vi "Sequence.vi"(8 "error in (no error)":errorcluster, 11 "Message Queues in":T65) -> (0 "error out":errorcluster)   [LabVIEW 2018, in "Sequencing Library.lvlib"]
uses:
  Sequencing Library.lvlib
  Main/Main Queue Cluster.ctl
  support/Message Queue/Message Cluster.ctl
  Drag and Drop/State Cluster.ctl
  Drag and Drop/Thumbnail Cluster.ctl
  Drag and Drop/Object Cluster.ctl
  <vilib>/Utility/miscctls.llb/LVRectTypeDef.ctl
  Drag and Drop/Object Type Enum.ctl
  <vilib>/Utility/miscctls.llb/LVPositionTypeDef.ctl
  Config Module/Controls/Main Config Cluster.ctl
  OPC/OPC Module Config.ctl
  Scale Module Folder/Measure Instrument/State Enum.ctl
  <vilib>/Utility/miscctls.llb/LVPoint32TypeDef.ctl
  OPC/OPC Settings.ctl
  OPC/Variable Data Cluster.ctl
  <vilib>/OPCUA/controls/NodeId.ctl
  <vilib>/OPCUA/controls/OPC UA StatusCode.ctl
  <vilib>/OPCUA/controls/Subscription ID.ctl
  <vilib>/OPCUA/controls/OPC UA Client Refnum.ctl
  <vilib>/OPCUA/controls/Subscription Data Change.ctl
  <vilib>/OPCUA/controls/Data Type.ctl
  Feed Module/Controls/Feed Module Config Cluster.ctl
  Feed Module/Controls/Feed Module Settings Cluster.ctl
  Ismatec ISM 831C/Controls/Ismatech Settings Cluster.ctl
  Masterflex 7550-30/Controls/Settings Cluster.ctl
  Mettler Toledo/Controls/Settings Cluster.ctl
  Bronkhorst M13 Flow Meter/Settings Cluster.ctl
  Measure Instrument/PID 2 Parameters Cluster.ctl
  Measure Instrument/PID Input Enum.ctl
  Measure Instrument/PID 2 Output Enum.ctl
  Tacmina QI/Tacmina QI DAQ Setting.ctl
  KNF Pump/Settings Cluster plus SIMDOS.ctl
  ASIA Pump/Pump Settings.ctl
  VICI M50 Party Mode/Settings Cluster.ctl
  FLOM Pump/Settings Cluster.ctl
  SSI PR Class/SSI PR or LD Settings Cluster.ctl
  Masterflex 75211/Masterflex 75211 DAQ Setting.ctl
  SSI PR Class/SSI P40 Settings Cluster.ctl
  TT Module/Controls/TT Module Config Cluster.ctl
  Tag VIs/Numeric Alarm Settings Cluster.ctl
  Acquisition/Hardware Configuration.ctl
  Acquisition/Task Cluster.ctl
  PT Module/Controls/PT Module Config Cluster.ctl
  Scale Module Folder/Feed Module/Controls/Scale Module Config Cluster.ctl
  Scale Module Folder/Feed Module/Controls/Scale Module Settings Cluster.ctl
  Pump Module Folder/Pump Module Config Cluster.ctl
  Pump Module Folder/Pump Module Settings Cluster.ctl
  LabJack Module/Controls/U3 Module Config Cluster.ctl
  Decoration Module/Decoration Module Config Cluster.ctl
  Flow Module Folder/Feed Module/Controls/Flow Module Config Cluster.ctl
  Flow Module Folder/Feed Module/Controls/Flow Module Settings Cluster.ctl
  TCU Module/TCU Module Folder/TCU Module Config Cluster.ctl
  TCU Module/TCU Module Folder/TCU Module Settings Cluster.ctl
  TCU Module/TCU Module Folder/Measure Instrument/Output Devices.ctl
  Huber TCU/Huber Settings.ctl
  Lauda Integral XT-150 TCU/Lauda Settings.ctl
  Julabo Type 1 TCU/Julabo Type 1 TCU Folder/Julabo FP-50 Settings.ctl
  Huber Unistat 410 TCU/Huber Unistat 410 RS485 Settings.ctl
  D-O Module Folder/Not Sure Where this is Used.ctl
  Squence Control.ctl
  D-O Module Folder/D-O Module Config Cluster.ctl
  D-O Module Folder/Valve Clusters.ctl
  D-O Module Folder/D-O Module Settings Cluster.ctl
  D-O Module Folder/D-O Device Settings Cluster.ctl
  VICI Electronic Actuator/VICI Electronic Actuator Settings.ctl
  Pressure Regulator Control Module/Pressure Regulator/Controls/4-20mA Module Config Cluster.ctl
  Pressure Regulator Control Module/Pressure Regulator/Controls/4-20mA Module Settings Cluster.ctl
  Pressure Transmitter/Pressure Transmitter Device Settings.ctl
  Pressure Reg Module/Pressure Regulator Device Settings.ctl
  Squence Update Cluster.ctl
  support/Message Queue/Enqueue Message (Single).vi
  support/Message Queue/Message Queue.lvlib
  support/Command Log VIs/Command Logging.lvlib
  Drag and Drop/Drag and Drop.lvlib
  Config Module/Config Module.lvlib
  TT Module/TT Module.lvlib
  Feed Module/Feed Module.lvlib
  Ismatec ISM 831C/Ismatec ISM 831C.lvlib
  Masterflex 7550-30/Masterflex 7550-30.lvlib
  Mettler Toledo/Mettler Toledo.lvlib
  Bronkhorst M13 Flow Meter/Bronkhorst M13 Flow Meter.lvlib
  Tacmina QI/Tacmina QI.lvlib
  KNF Pump/KNF SIMDOS.lvlib
  ASIA Pump.lvlib
  DAQ/DAQ.lvlib
  PT Module/PT Module.lvlib
  Scale Module Folder/Scale Module.lvlib
  Pump Module Folder/Pump Module.lvlib
  LabJack Module/U3 Module.lvlib
  Flow Module Folder/Flow Module.lvlib
  TCU Module/TCU Module Folder/TCU Module.lvlib
  Huber TCU/Huber Ministat 230 TCU.lvlib
  Lauda Integral XT-150 TCU/Lauda TCU.lvlib
  Julabo Type 1 TCU/Julabo Type 1 TCU Folder/Julabo Type FP-50 TCU.lvlib
  VICI M50 Party Mode/VICI M6 M50 Party Mode.lvlib
  D-O Module Folder/D-O Module.lvlib
  Pressure Transmitter/Pressure Transmitter Library.lvlib
  Pressure Regulator Control Module/Pressure Regulator/4-20mA Module.lvlib
  Pressure Reg Module/Pressure Regulator Library.lvlib
  FLOM Pump/FLOM Pump.lvlib
  SSI PR Class/SSI PR or LD Pump.lvlib
  OPC/OPC UA.lvlib
  Scale Module Folder/Measure Instrument/Scale Module Engine.lvlib
  D-O Module Folder/DIO Valve/VICI Electronic Actuator.lvlib
  Masterflex 75211/Masterflex 75211.lvlib
  SSI PR Class/SSI P40 Pump.lvlib
  Huber Unistat 410 TCU/Huber Unistat 410 TCU.lvlib
panel:
  out "Metrics:Code Size":u32
  out "Metrics:Total Data Size":u32
  out "Application:All VIs In Memory":string[](array[string])
  out "error out 2":errorcluster
  out "Process Name":string
  out "Queue Name":string
  out "Loop Variable":u32
  out "Step":i32
  out "Done":bool
  out "Output":T1 {"Main Config"."PR Module Configs"."Settings"."PID 2 Parameters"."output range"."output low" format="%.2f"; "Main Config"."PR Module Configs"."Settings"."PID 2 Parameters"."output range"."output high" min=0.0 max=100.0 format="%.2f"; "Main Config"."PR Module Configs"."Settings"."PID 2 Parameters"."PID gains"."derivative time (Td, min)" format="%.3f"; "Main Config"."PR Module Configs"."Settings"."PID 2 Parameters"."PID gains"."integral time (Ti, min)" format="%.3f"; "Main Config"."PR Module Configs"."Settings"."PID 2 Parameters"."PID gains"."proportional gain (Kc)" format="%.3f"; "Main Config"."Steps"."Control" items=["Pump %", "Setpoint"]; "Main Config"."TCU Module Configs"."Settings"."Huber Unistat 410 Settings"."Address" min=0 max=99 format="%02.0f"; "Main Config"."TCU Module Configs"."Settings"."Julabo FP-50 Settings"."Pump Power" min=0 max=8 step=1; "Main Config"."TCU Module Configs"."Settings"."Lauda Settings"."Pump Power" min=0 max=8 step=1; "Main Config"."Pump Module Configs"."Settings"."ASIA Pump C"."channel" min=0 max=1 step=1; "Main Config"."Pump Module Configs"."Settings"."Masterflex"."Pump Number" min=1.0 max=20.0 step=1.0; "Main Config"."Pump Module Configs"."Settings"."Ismatech"."Pump Number" min=1.0 max=20.0 step=1.0; "Main Config"."Feed Module Configs"."Settings"."output range"."output low" min=0.0 max=100.0 format="%.2f"; "Main Config"."Feed Module Configs"."Settings"."output range"."output high" format="%.2f"; "Main Config"."Feed Module Configs"."Settings"."PID 2 Parameters"."PID gains"."derivative time (Td, min)" format="%.3f"; "Main Config"."Feed Module Configs"."Settings"."PID 2 Parameters"."PID gains"."integral time (Ti, min)" format="%.3f"; "Main Config"."Feed Module Configs"."Settings"."PID 2 Parameters"."PID gains"."proportional gain (Kc)" format="%.3f"; "Main Config"."Feed Module Configs"."Settings"."ASIA Pump C"."channel" min=0 max=1 step=1; "Main Config"."Feed Module Configs"."Settings"."Ismatech"."Pump Number" min=1.0 max=20.0 step=1.0; "Main Config"."Feed Module Configs"."Settings"."Masterflex"."Pump Number" min=1.0 max=20.0 step=1.0}
  out "Intruction Cluster":T55 {"Control" items=["Setpoint", "Pump %"]}
  out "Paused":bool
  out "Stop":bool
  in  "Input":T1 {"Main Config"."PR Module Configs"."Settings"."PID 2 Parameters"."output range"."output low" format="%.2f"; "Main Config"."PR Module Configs"."Settings"."PID 2 Parameters"."output range"."output high" min=0.0 max=100.0 format="%.2f"; "Main Config"."PR Module Configs"."Settings"."PID 2 Parameters"."PID gains"."derivative time (Td, min)" format="%.3f"; "Main Config"."PR Module Configs"."Settings"."PID 2 Parameters"."PID gains"."integral time (Ti, min)" format="%.3f"; "Main Config"."PR Module Configs"."Settings"."PID 2 Parameters"."PID gains"."proportional gain (Kc)" format="%.3f"; "Main Config"."Steps"."Control" items=["Pump %", "Setpoint"]; "Main Config"."TCU Module Configs"."Settings"."Huber Unistat 410 Settings"."Address" min=0 max=99 format="%02.0f"; "Main Config"."TCU Module Configs"."Settings"."Julabo FP-50 Settings"."Pump Power" min=0 max=8 step=1; "Main Config"."TCU Module Configs"."Settings"."Lauda Settings"."Pump Power" min=0 max=8 step=1; "Main Config"."Pump Module Configs"."Settings"."ASIA Pump C"."channel" min=0 max=1 step=1; "Main Config"."Pump Module Configs"."Settings"."Masterflex"."Pump Number" min=1.0 max=20.0 step=1.0; "Main Config"."Pump Module Configs"."Settings"."Ismatech"."Pump Number" min=1.0 max=20.0 step=1.0; "Main Config"."Feed Module Configs"."Settings"."output range"."output low" min=0.0 max=100.0 format="%.2f"; "Main Config"."Feed Module Configs"."Settings"."output range"."output high" format="%.2f"; "Main Config"."Feed Module Configs"."Settings"."PID 2 Parameters"."PID gains"."derivative time (Td, min)" format="%.3f"; "Main Config"."Feed Module Configs"."Settings"."PID 2 Parameters"."PID gains"."integral time (Ti, min)" format="%.3f"; "Main Config"."Feed Module Configs"."Settings"."PID 2 Parameters"."PID gains"."proportional gain (Kc)" format="%.3f"; "Main Config"."Feed Module Configs"."Settings"."ASIA Pump C"."channel" min=0 max=1 step=1; "Main Config"."Feed Module Configs"."Settings"."Ismatech"."Pump Number" min=1.0 max=20.0 step=1.0; "Main Config"."Feed Module Configs"."Settings"."Masterflex"."Pump Number" min=1.0 max=20.0 step=1.0}
  # "Instrument Settings"
  # "Instrument Settings"
  # "Output Instruments"
  # "Flow Meter Settings"
  # "Output Instruments"
  # "Scale Settings"
  # "Output Instruments"
  # "Input Instruments"
  # "Instrument Settings"
  # "Instrument Settings"
  # "Output Instruments"
  # "Flow Meter Settings"
  # "Output Instruments"
  # "Scale Settings"
  # "Output Instruments"
  # "Input Instruments"
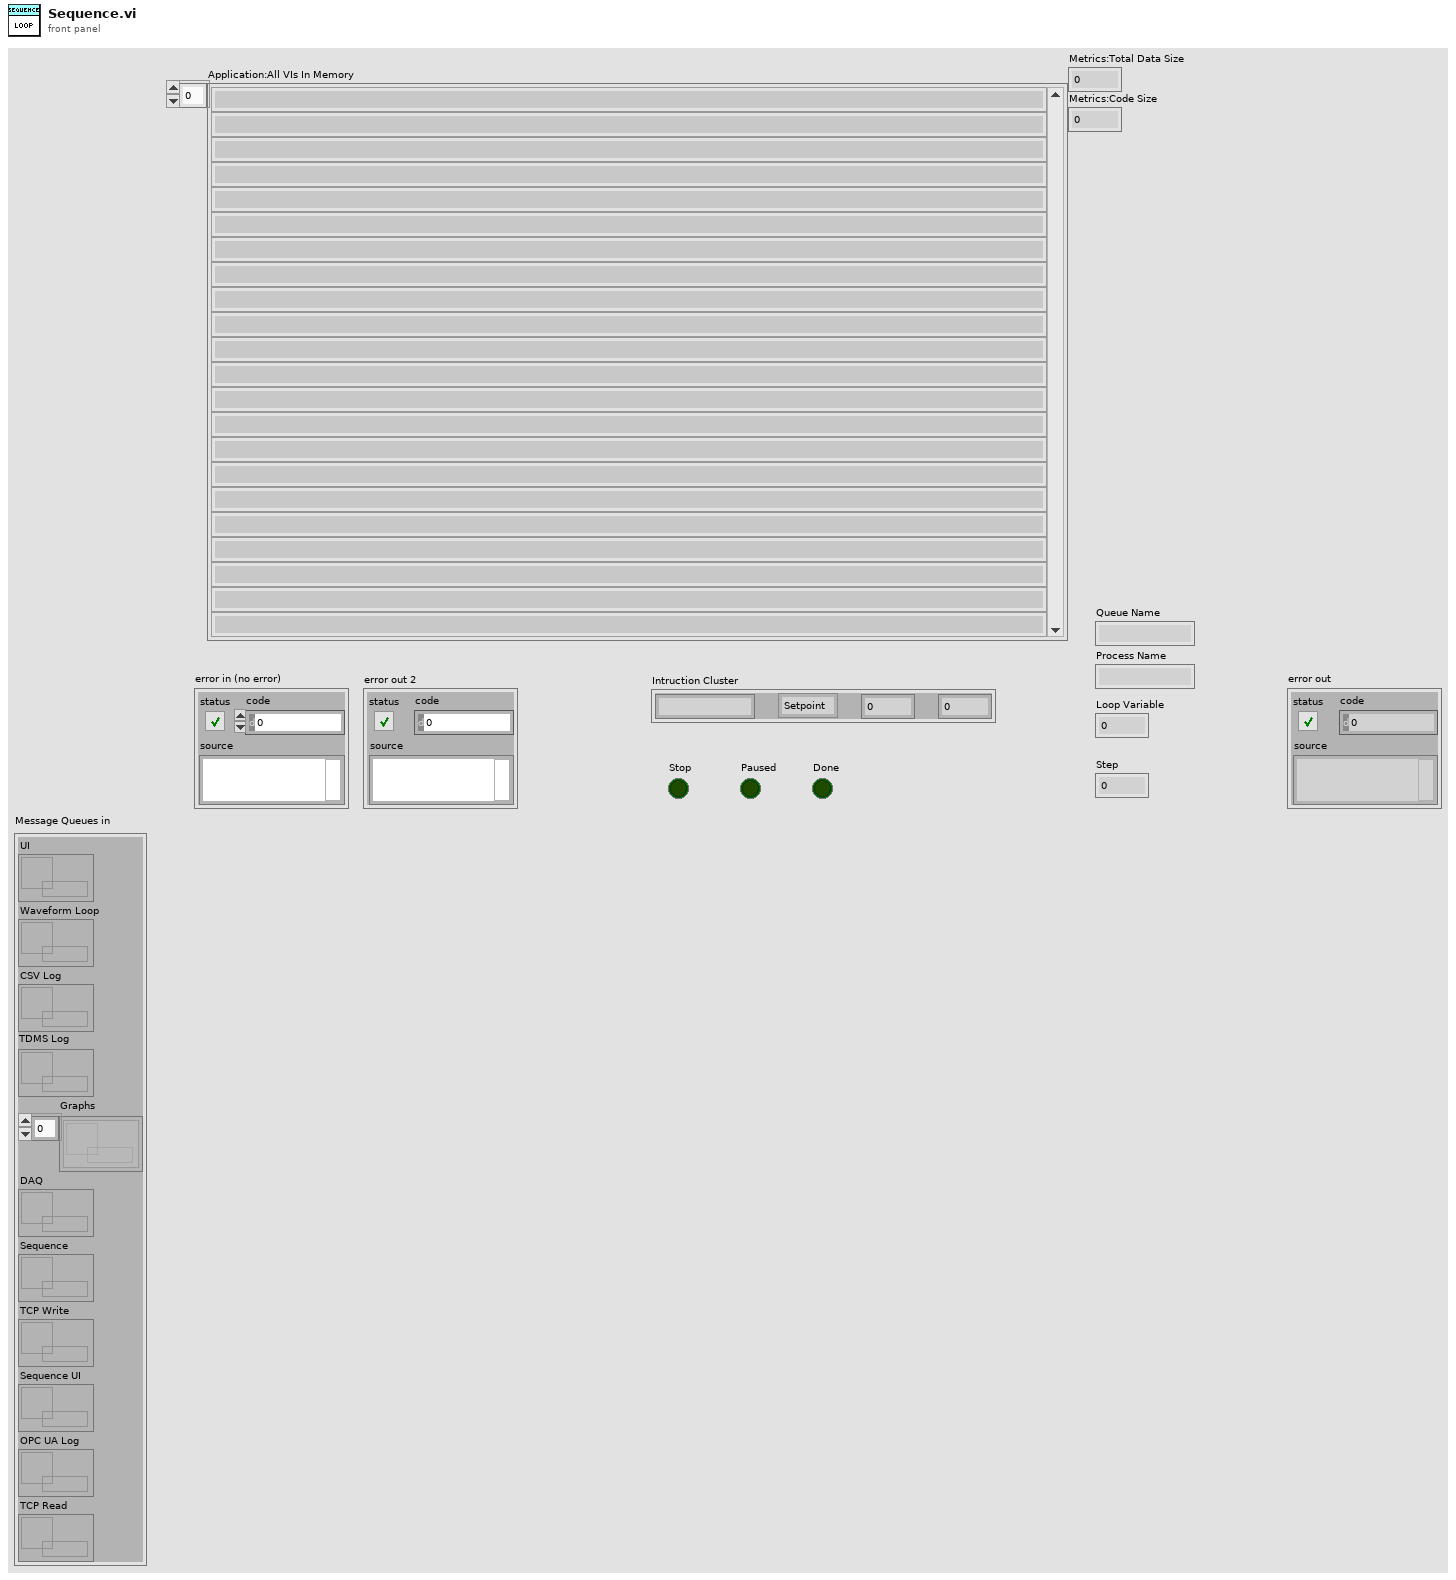
[diagram p1: front panel]
types:
  T1 = typedef "Drag and Drop.lvlib/State Cluster.ctl" = cluster{"VI refs":refnum<vi>[], "Queues":refnum<queue>[], "[Thumbnails]":T2[], "Drag Object Idx":i32, "[Objects]":T3[], "Active Object":i32, "Drop Offset":T6, "Process Name":string, "Main Config":T7, "Campaign Filepath":path, "Config Changed?":bool}
  T2 = typedef "Thumbnail Cluster.ctl" = cluster{"Path":path, "Rectangle":cluster{"left":i16, "top":i16, "right":i16, "bottom":i16}}
  T3 = typedef "Object Cluster.ctl" = cluster{"BMP Path":path, "Anchor Position":cluster{"X":i32, "Y":i32}, "Hot Spot":T4, "Type":T5, "Parameters":variant}
  T4 = typedef "LVRectTypeDef.ctl" = cluster{"Left":i16, "Top":i16, "Right":i16, "Bottom":i16}
  T5 = typedef "Object Type Enum.ctl" = enum16{"Icon", "Line", "Text", "Feed Module"}
  T6 = typedef "LVPositionTypeDef.ctl" = cluster{"Left":i32, "Top":i32}
  T7 = typedef "Config Module.lvlib/Main Config Cluster.ctl" = cluster{"Notebook":string, "Page":string, "OPC Module Configs":T8[], "Feed Module Configs":T17[], "Log File Path":path, "TT Module Configs":T34[], "DAQ Config":T36, "PT Module Configs":T38[], "Scale Module Configs":T39[], "Pump Module Configs":T41[], "U3 Module Configs":T43[], "Decoration Module Configs":T44[], "Flow Module Configs":T45[], "TCU Module Configs":T47[], "Steps":T54, "Abort":bool, "DO Module Configs":T56[], "PR Module Configs":T61[], "Cycle Period":dbl}
  T8 = typedef "OPC UA.lvlib/OPC Module Config.ctl" = cluster{"State":T9, "GUID":string, "Drop Coords":T10, "Configuration":T11, "First Iteration":bool, "Data":cluster{"Object Name":string, "Variable Array":T12[]}[], "Process Name":string, "Load Count":i32, "Log Started":bool, "subscription ID out":T15, "OPC UA client refnum out":T16, "Event Registration Refnum":refnum<event-registration>, "Start Time":timestamp, "Current Time":timestamp}
  T9 = typedef "Scale Module.lvlib/Scale Module Engine.lvlib/State Enum.ctl" = enum16{"Measuring", "Idle"}
  T10 = typedef "LVPoint32TypeDef.ctl" = cluster{"Horizontal":i32, "Vertical":i32}
  T11 = typedef "OPC UA.lvlib/OPC Settings.ctl" = cluster{"Cycle Period":dbl, "server endpoint URL":string, "security policy":cluster{"message mode":enum16{"None", "Sign", "Sign and Encrypt"}, "security":enum16{"Basic256", "Basic128Rsa15"}}, "Trust Any Server":bool}
  T12 = typedef "OPC UA.lvlib/Variable Data Cluster.ctl" = cluster{"node ID":T13, "browse name":string, "status":T14, "timestamp":timestamp, "value ":variant}
  T13 = typedef "NodeId.ctl" = string
  T14 = typedef "OPC UA StatusCode.ctl" = u32
  T15 = typedef "Subscription ID.ctl" = u32
  T16 = typedef "OPC UA Client Refnum.ctl" = refnum<k21>
  T17 = typedef "Feed Module.lvlib/Feed Module Config Cluster.ctl" = cluster{"GUID":string, "Drop Coords":T10, "Process Name":string, "Queue Name":string, "Settings":T18, "Settings Load Count":i32, "OP Load Count":i32}
  T18 = typedef "Feed Module.lvlib/Feed Module Settings Cluster.ctl" = cluster{"Cycle Period":dbl, "Ismatech":T19, "Masterflex":T20, "Mettler":T21, "Bronkhorst M13 Flow Meter":T22, "PID 2 Parameters":T23, "Manual Entry":dbl, "Auto?":bool, "output range":cluster{"output high":dbl, "output low":dbl}, "Bronkhorst M14":T21, "Tacmina Settings":T26, "KNF SIMDOS Settings":T27, "ASIA Pump C":T28, "VICI Settings":T29, "FLOM Settings":T30, "SSI PR/LD Settings":T31, "Masterflex 75211 Settings":T32, "SSI P40 Settings":T33}
  T19 = typedef "Ismatec ISM 831C.lvlib/Ismatech Settings Cluster.ctl" = cluster{"VISA resource name":refnum<visa-resource-name>, "Simulated?":bool, "Pump Number":dbl, "Reverse?":bool}
  T20 = typedef "Masterflex 7550-30.lvlib/Settings Cluster.ctl" = cluster{"VISA resource name":refnum<visa-resource-name>, "Simulated?":bool, "Pump Number":dbl, "Reverse?":bool}
  T21 = typedef "Mettler Toledo.lvlib/Settings Cluster.ctl" = cluster{"VISA resource name":refnum<visa-resource-name>, "Simulated?":bool}
  T22 = typedef "Bronkhorst M13 Flow Meter.lvlib/Settings Cluster.ctl" = cluster{"VISA resource name":refnum<visa-resource-name>, "Simulated?":bool}
  T23 = typedef "PID 2 Parameters Cluster.ctl" = cluster{"Input Device":T24, "Output Device":T25, "Setpoint":dbl, "PID gains":cluster{"proportional gain (Kc)":dbl, "integral time (Ti, min)":dbl, "derivative time (Td, min)":dbl}}
  T24 = typedef "PID Input Enum.ctl" = enum16{"Default", "Bronkhorst M13", "Bronkhorst M14", "Scale Rate of Change"}
  T25 = typedef "PID 2 Output Enum.ctl" = enum16{"Default", "Ismatec ISM 831C", "Masterflex 7550-30", "VICI", "Tacmina QI", "KNF SIMDOS", "ASIA Type C", "FLOM UI-22-11", "SSI PR/LD", "SSI P40", "Masterflex 75211-70"}
  T26 = typedef "Tacmina QI.lvlib/Tacmina QI DAQ Setting.ctl" = cluster{"Analog DAQ Task":refnum<k21>, "Digital DAQ Task":refnum<k21>}
  T27 = typedef "KNF SIMDOS.lvlib/Settings Cluster plus SIMDOS.ctl" = cluster{"VISA resource name":refnum<visa-resource-name>, "Simulated?":bool}
  T28 = typedef "ASIA Pump.lvlib/Pump Settings.ctl" = cluster{"ASIA Pump #":i32, "channel":i32, "Simulated":bool}
  T29 = typedef "VICI M6 M50 Party Mode.lvlib/Settings Cluster.ctl" = cluster{"VISA resource name":refnum<visa-resource-name>, "Simulated?":bool, "Pump Letter":string, "Reverse?":bool}
  T30 = typedef "FLOM Pump.lvlib/Settings Cluster.ctl" = cluster{"VISA resource name":refnum<visa-resource-name>, "Simulated?":bool, "Pump Number":dbl}
  T31 = typedef "SSI PR or LD Pump.lvlib/SSI PR or LD Settings Cluster.ctl" = cluster{"VISA resource name":refnum<visa-resource-name>, "Simulated?":bool}
  T32 = typedef "Masterflex 75211.lvlib/Masterflex 75211 DAQ Setting.ctl" = cluster{"Analog DAQ Task":refnum<k21>, "Digital DAQ Task":refnum<k21>}
  T33 = typedef "SSI P40 Pump.lvlib/SSI P40 Settings Cluster.ctl" = cluster{"VISA resource name":refnum<visa-resource-name>, "Simulated?":bool}
  T34 = typedef "TT Module.lvlib/TT Module Config Cluster.ctl" = cluster{"GUID":string, "Drop Coords":T10, "Input Channel Tag Name ":string, "Process Name":string, "Queue Name":string, "Input Channel Numeric Alarm Settings":T35[]}
  T35 = typedef "Numeric Alarm Settings Cluster.ctl" = cluster{"enable? (F)":bool, "name":string, "alarm type":enum16{"HI_HI", "HI", "LO", "LO_LO"}, "level/change":dbl, "deadband/time":dbl, "alarm delay":dbl, "priority":u32, "ack type":enum16{"Auto", "User", "None", "Each Occurrence"}, "area":string, "description":string, "log? (T)":bool}
  T36 = typedef "DAQ.lvlib/Hardware Configuration.ctl" = cluster{"Tasks":T37[]}
  T37 = typedef "Task Cluster.ctl" = cluster{"DAQmx Task":refnum<k21>, "Read-Write Radio":enum32{"Read", "Write"}}
  T38 = typedef "PT Module.lvlib/PT Module Config Cluster.ctl" = cluster{"GUID":string, "Drop Coords":T10, "Input Channel Tag Name ":string, "Process Name":string, "Queue Name":string, "Input Channel Numeric Alarm Settings":T35[]}
  T39 = typedef "Scale Module.lvlib/Scale Module Config Cluster.ctl" = cluster{"GUID":string, "Drop Coords":T10, "Process Name":string, "Queue Name":string, "Settings":T40, "Load Count":i32}
  T40 = typedef "Scale Module.lvlib/Scale Module Settings Cluster.ctl" = cluster{"Cycle Period":dbl, "Mettler":T21, "Scale Type":string}
  T41 = typedef "Pump Module.lvlib/Pump Module Config Cluster.ctl" = cluster{"GUID":string, "Drop Coords":T10, "Process Name":string, "Queue Name":string, "Settings":T42, "Load Count":i32}
  T42 = typedef "Pump Module.lvlib/Pump Module Settings Cluster.ctl" = cluster{"Cycle Period":dbl, "Manual Entry":dbl, "Output Device":T25, "Ismatech":T19, "Masterflex":T20, "VICI Settings":T29, "Tacmina Settings":T26, "KNF SIMDOS Settings":T27, "ASIA Pump C":T28, "FLOM Settings":T30, "SSI PR/LD Settings":T31, "SSI P40 Settings":T31, "Masterflex 75211 Settings":T32, "Pump Calibration File":path, "Calibration Slope":dbl, "Calibration Y Intercept":dbl, "Pump Cal Enum":u16}
  T43 = typedef "U3 Module.lvlib/U3 Module Config Cluster.ctl" = cluster{"GUID":string, "Drop Coords":T10, "AI Channel Number":enum16{"Default", "AI0", "AI1", "AI2", "AI3", "AI4", "AI5", "AI6", "AI7"}, "Process Name":string, "Queue Name":string, "Input Channel Numeric Alarm Settings":T35[]}
  T44 = typedef "Decoration Module Config Cluster.ctl" = cluster{"GUID":string, "Drop Coords":T10, "Decoration Filepath":path}
  T45 = typedef "Flow Module.lvlib/Flow Module Config Cluster.ctl" = cluster{"GUID":string, "Drop Coords":T10, "Process Name":string, "Queue Name":string, "Settings":T46, "Load Count":i32}
  T46 = typedef "Flow Module.lvlib/Flow Module Settings Cluster.ctl" = cluster{"Cycle Period":dbl, "Bronkhorst M13":T21, "Flow Meter Type":string, "Bronkhorst M14":T21}
  T47 = typedef "TCU Module.lvlib/TCU Module Config Cluster.ctl" = cluster{"GUID":string, "Drop Coords":T10, "Process Name":string, "Queue Name":string, "Settings":T48, "Load Count":i32, "Power Level Changed":bool}
  T48 = typedef "TCU Module.lvlib/TCU Module Settings Cluster.ctl" = cluster{"Cycle Period":dbl, "Setpoint Entry":dbl, "Output Device":T49, "Huber Ministat 230 Settings":T50, "Lauda Settings":T51, "Julabo FP-50 Settings":T52, "Internal Control?":bool, "Huber Unistat 410 Settings":T53}
  T49 = typedef "Output Devices.ctl" = enum16{"Default", "Huber Ministat 230", "Huber Unistat 410", "Lauda XT-150", "Julabo FP-50"}
  T50 = typedef "Huber Ministat 230 TCU.lvlib/Huber Settings.ctl" = cluster{"VISA resource name":refnum<visa-resource-name>, "Simulated?":bool}
  T51 = typedef "Lauda TCU.lvlib/Lauda Settings.ctl" = cluster{"VISA resource name":refnum<visa-resource-name>, "Simulated?":bool, "Pump Power":i32}
  T52 = typedef "Julabo Type FP-50 TCU.lvlib/Julabo FP-50 Settings.ctl" = cluster{"VISA resource name":refnum<visa-resource-name>, "Simulated?":bool, "Pump Power":i32}
  T53 = typedef "Huber Unistat 410 TCU.lvlib/Huber Unistat 410 RS485 Settings.ctl" = cluster{"VISA resource name":refnum<visa-resource-name>, "Address":i8, "Simulated?":bool}
  T54 = typedef "Not Sure Where this is Used.ctl" = T55[]
  T55 = typedef "Sequencing Library.lvlib/Squence Control.ctl" = cluster{"Module":string, "Control":u16, "Value":dbl, "Wait (sec)":dbl}
  T56 = typedef "D-O Module.lvlib/D-O Module Config Cluster.ctl" = cluster{"GUID":string, "Drop Coords":T10, "Process Name":string, "Queue Name":string, "Settings":T57, "Load Count":i32}
  T57 = typedef "D-O Module.lvlib/Valve Clusters.ctl" = cluster{"Valve Settings":T58, "Valve Type":enum16{"Default", "Digital Output Valve", "VICI Electronic Actuator"}, "Time On (Sec)":dbl, "Time Off (Sec)":dbl, "Run?":bool}
  T58 = typedef "D-O Module.lvlib/D-O Module Settings Cluster.ctl" = cluster{"D-O Settings":T59, "VICI Electronic Actuator":T60}
  T59 = typedef "D-O Module.lvlib/D-O Device Settings Cluster.ctl" = cluster{"DAQmx Task Name":refnum<k21>, "Output Channel":u16, "Output Channel Names":string[]}
  T60 = typedef "VICI Electronic Actuator.lvlib/VICI Electronic Actuator Settings.ctl" = cluster{"VISA resource name":refnum<visa-resource-name>, "Mode":enum16{"Two Positions With Stops", "Two Positions Without Stops", "Mutiposition"}, "Simulated":bool}
  T61 = typedef "4-20mA Module.lvlib/4-20mA Module Config Cluster.ctl" = cluster{"GUID":string, "Drop Coords":T10, "Process Name":string, "Queue Name":string, "Settings":T62, "Settings Load Count":i32}
  T62 = typedef "4-20mA Module.lvlib/4-20mA Module Settings Cluster.ctl" = cluster{"Cycle Period":dbl, "PID 2 Parameters":cluster{"Input Device":enum16{"Default", "4-20mA"}, "Output Device":enum16{"Default", "Equilibar Pressure Reg", "Flow Regulator"}, "Setpoint":dbl, "PID gains":cluster{"proportional gain (Kc)":dbl, "integral time (Ti, min)":dbl, "derivative time (Td, min)":dbl}, "output range":cluster{"output low":dbl, "output high":dbl}}, "Manual Entry":dbl, "Auto?":bool, "4-20mA Input Settings":T63, "4-20mA Out Settings":T64, "Input Channel Tag Name ":string}
  T63 = typedef "Pressure Transmitter Library.lvlib/Pressure Transmitter Device Settings.ctl" = cluster{"Input Channel ":u16}
  T64 = typedef "Pressure Regulator Library.lvlib/Pressure Regulator Device Settings.ctl" = cluster{"Output DAQ Task":refnum<k21>}
  T65 = typedef "Main Queue Cluster.ctl" = cluster{"UI":refnum<queue>, "Waveform Loop":refnum<queue>, "CSV Log":refnum<queue>, "TDMS Log":refnum<queue>, "Graphs":refnum<queue>[], "DAQ":refnum<queue>, "Sequence":refnum<queue>, "TCP Write":refnum<queue>, "Sequence UI":refnum<queue>, "OPC UA Log":refnum<queue>, "TCP Read":refnum<queue>}
  T66 = typedef "Sequencing Library.lvlib/Squence Update Cluster.ctl" = cluster{"Auto?":bool, "Manual Entry":dbl, "Setpoint":dbl}
  T67 = enum16{"open", "replace", "create", "open or create", "replace or create", "replace or create with confirmation"}
  T68 = typedef "Support Library.lvlib/Message Queue.lvlib/Message Cluster.ctl" = cluster{"Message":string, "Message Data":variant}
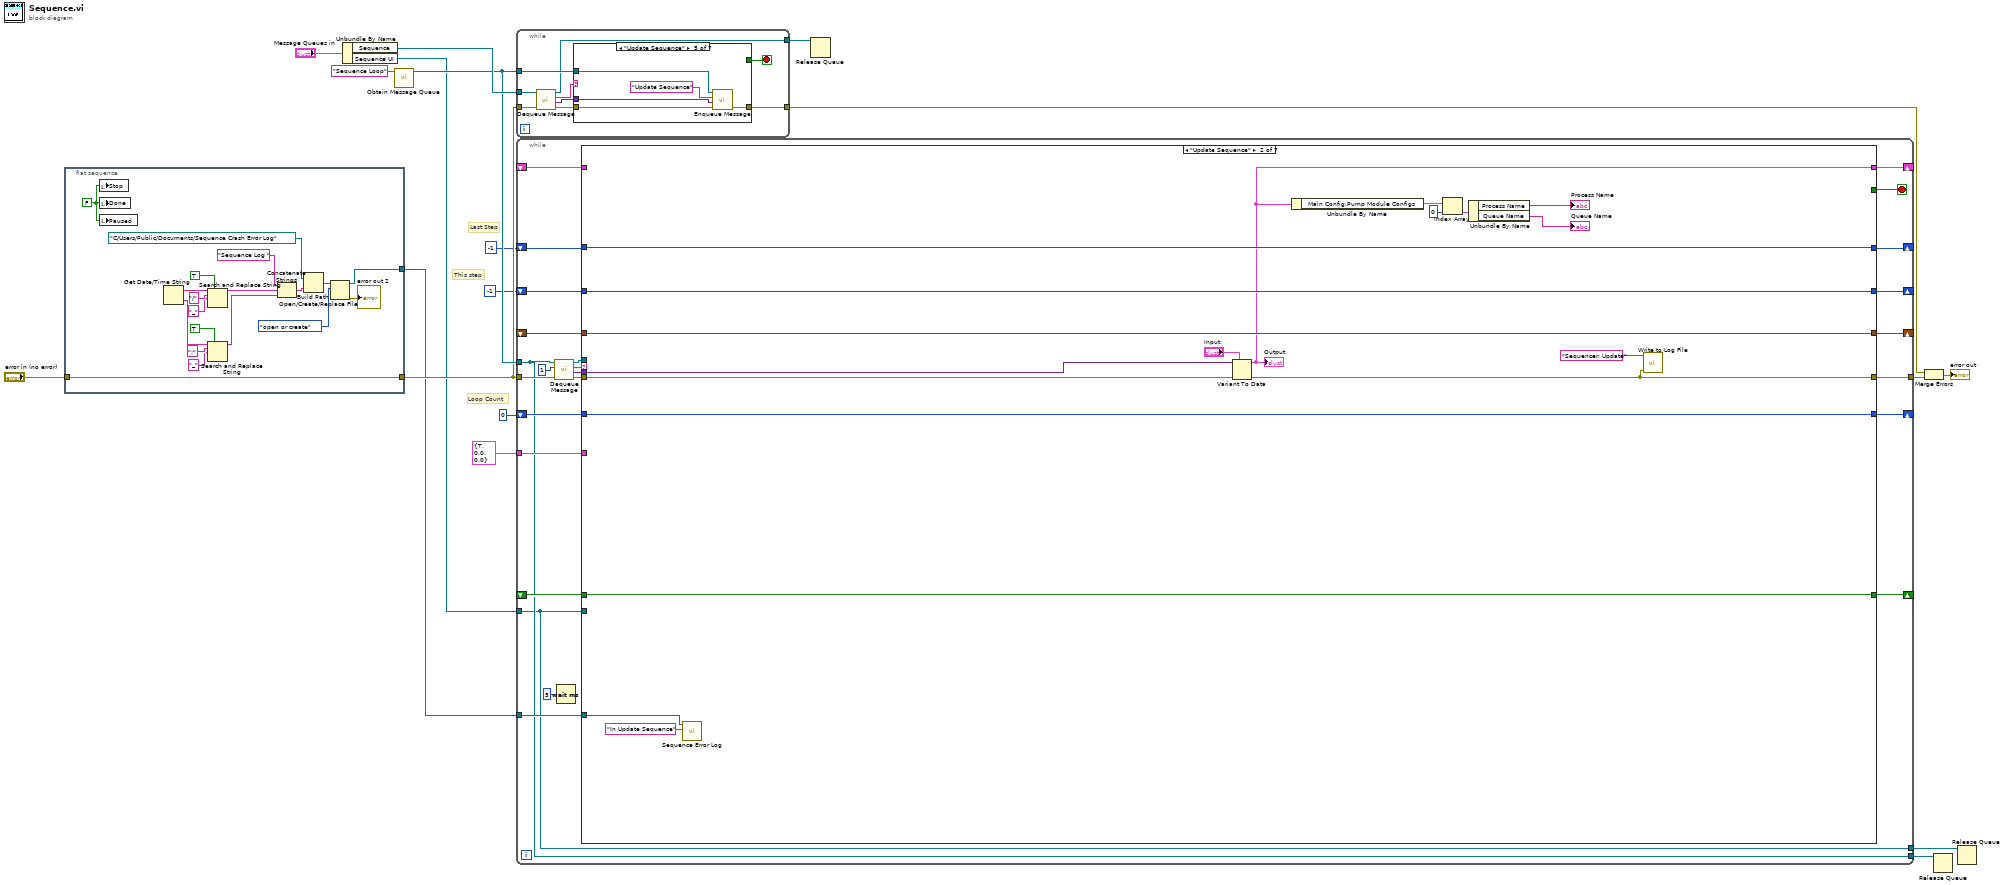
[diagram p0: block diagram]
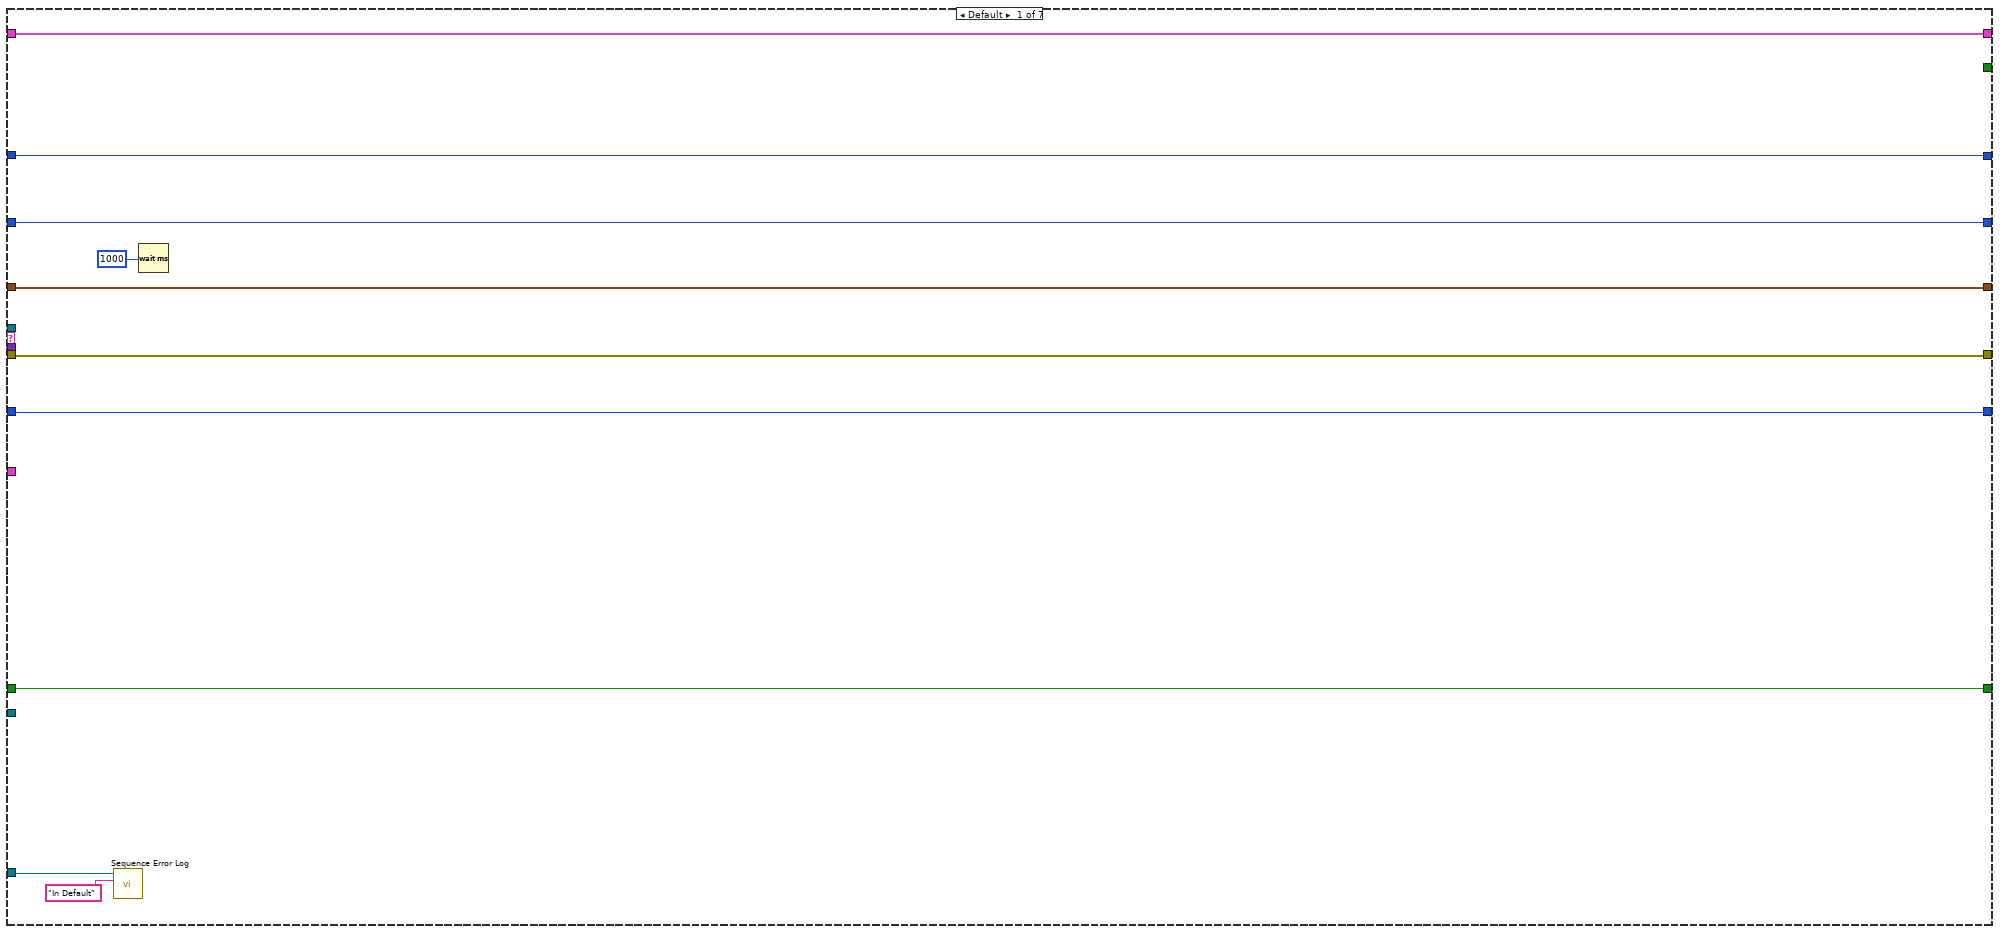
[diagram p2: hidden frame]
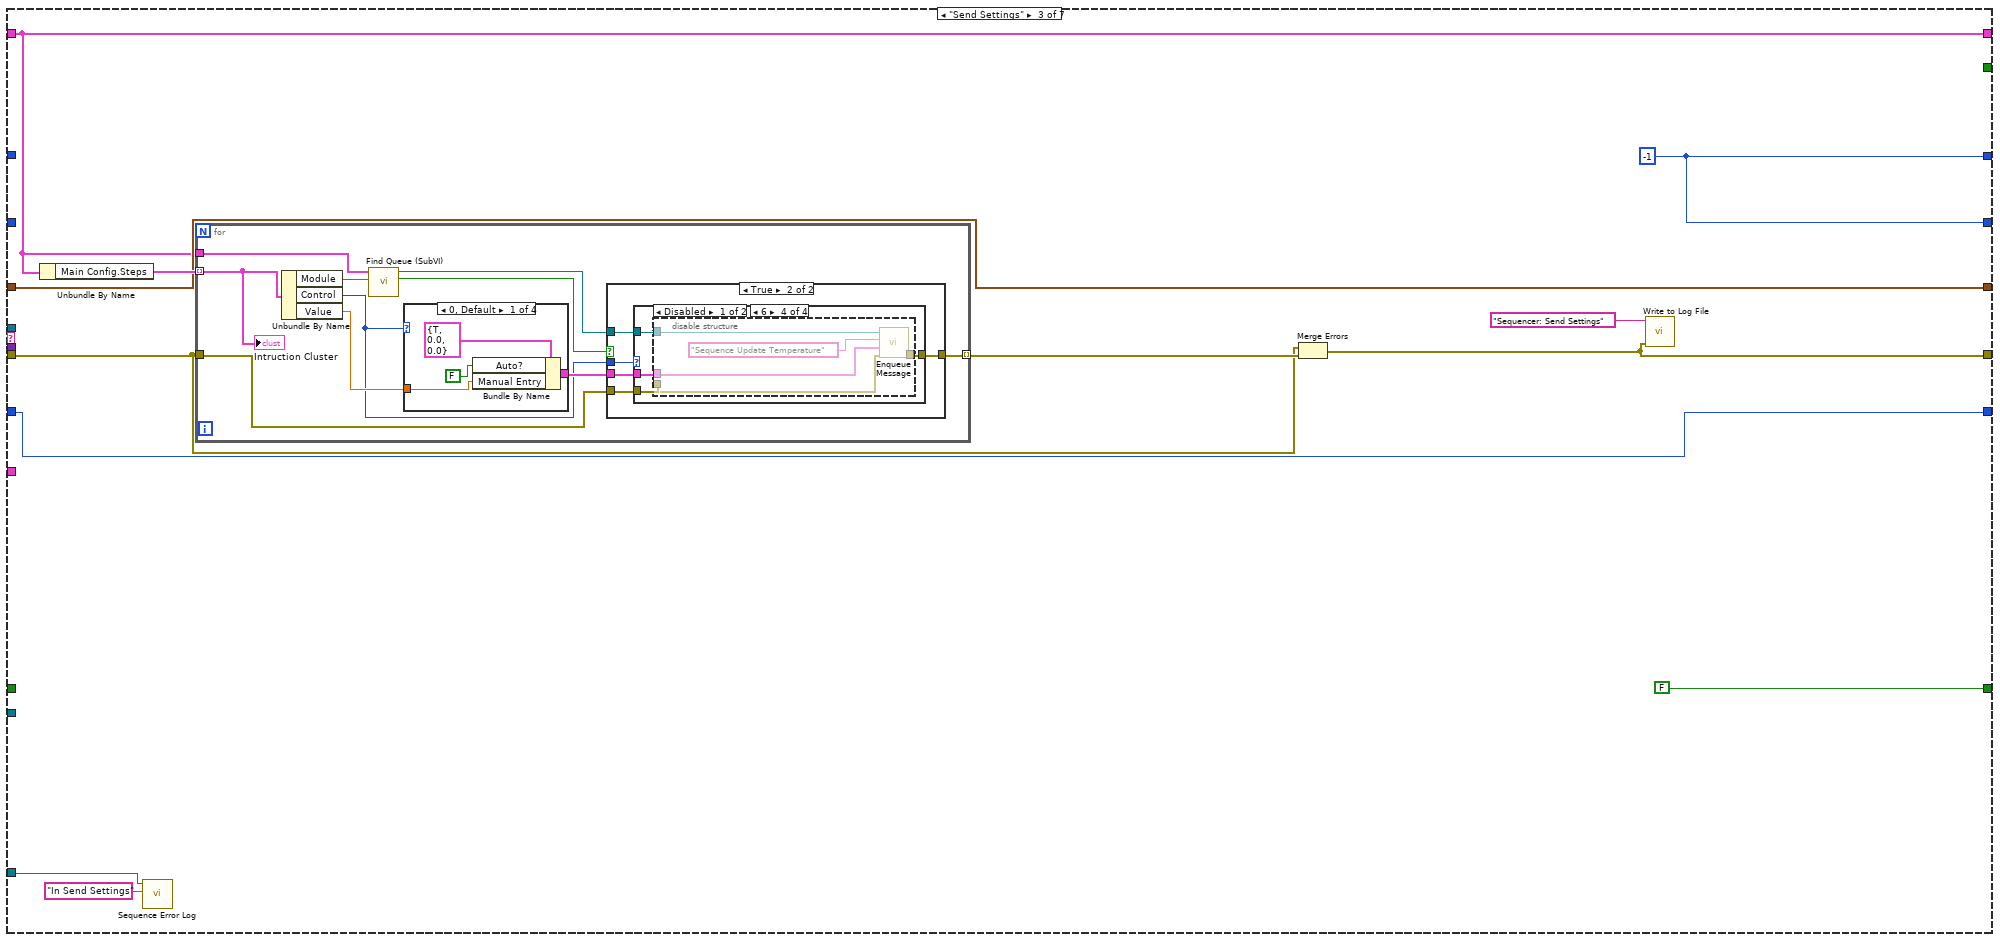
[diagram p3: hidden frame]
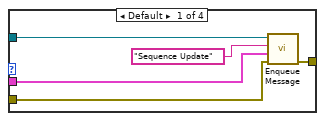
[diagram p5: hidden frame]
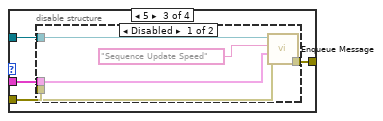
[diagram p7: hidden frame]
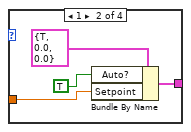
[diagram p10: hidden frame]
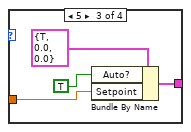
[diagram p11: hidden frame]
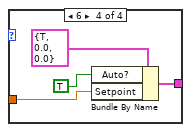
[diagram p12: hidden frame]
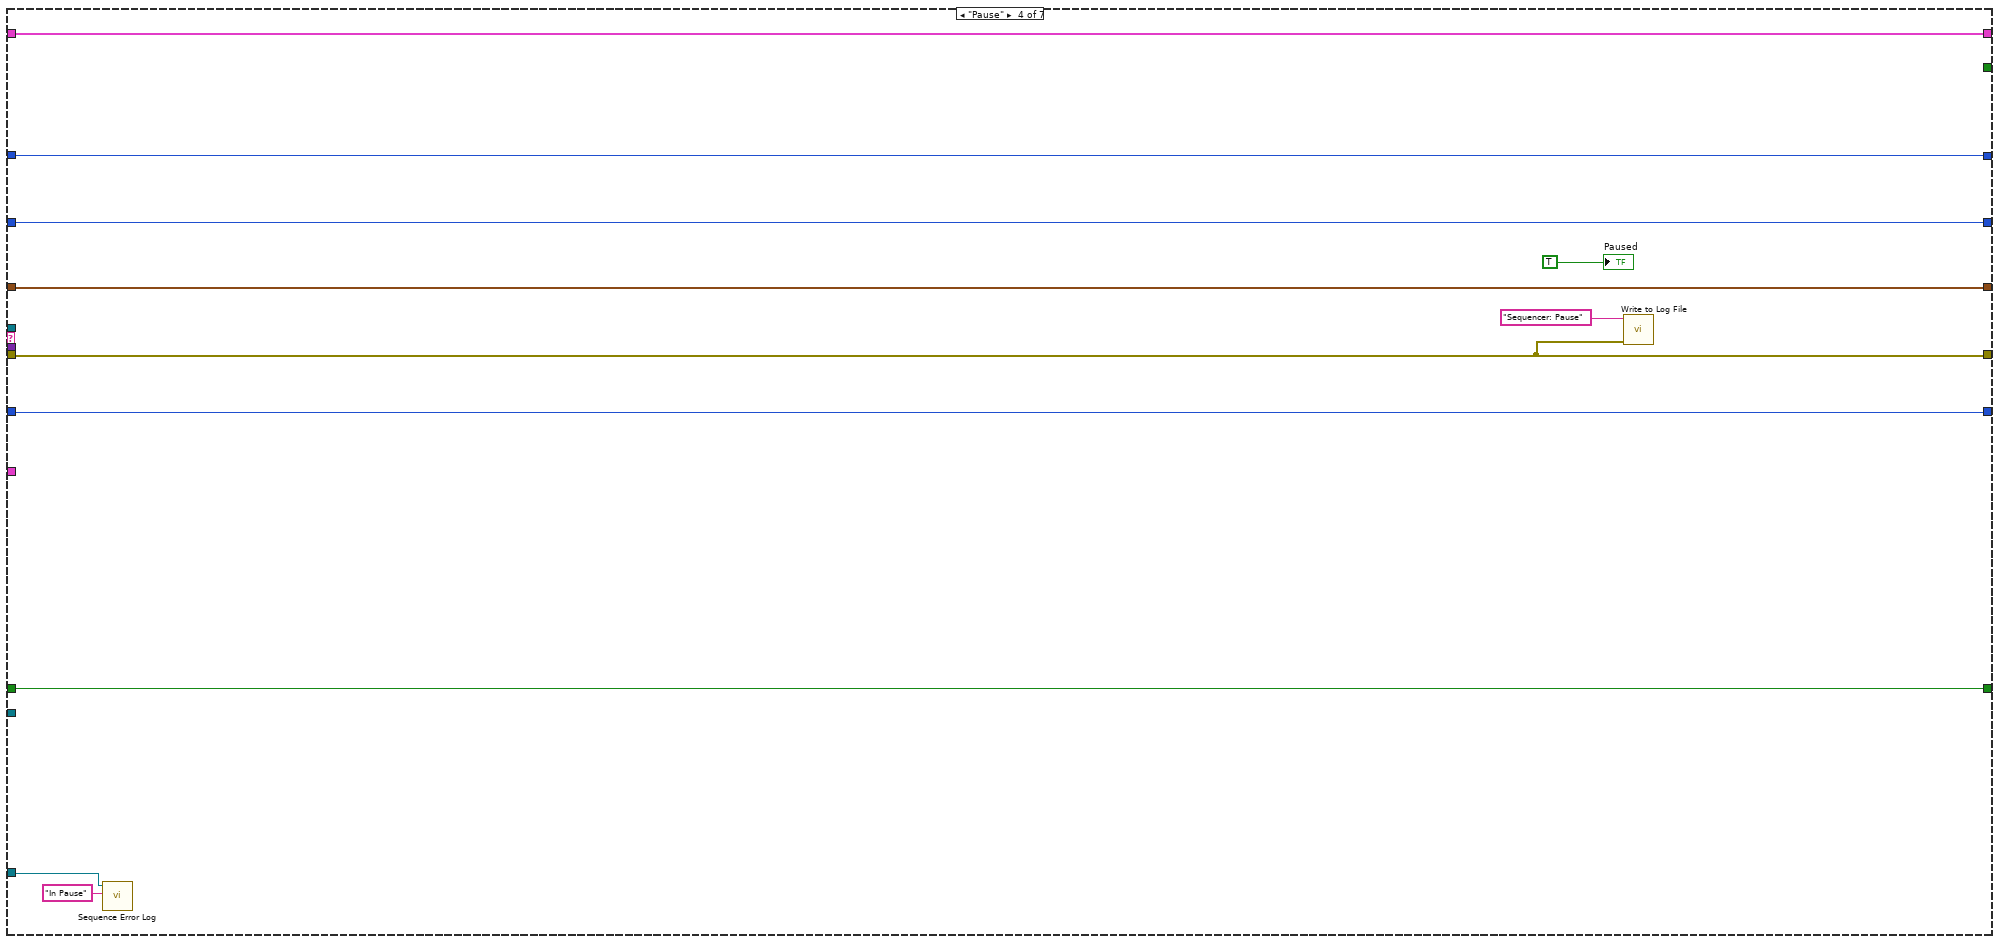
[diagram p13: hidden frame]
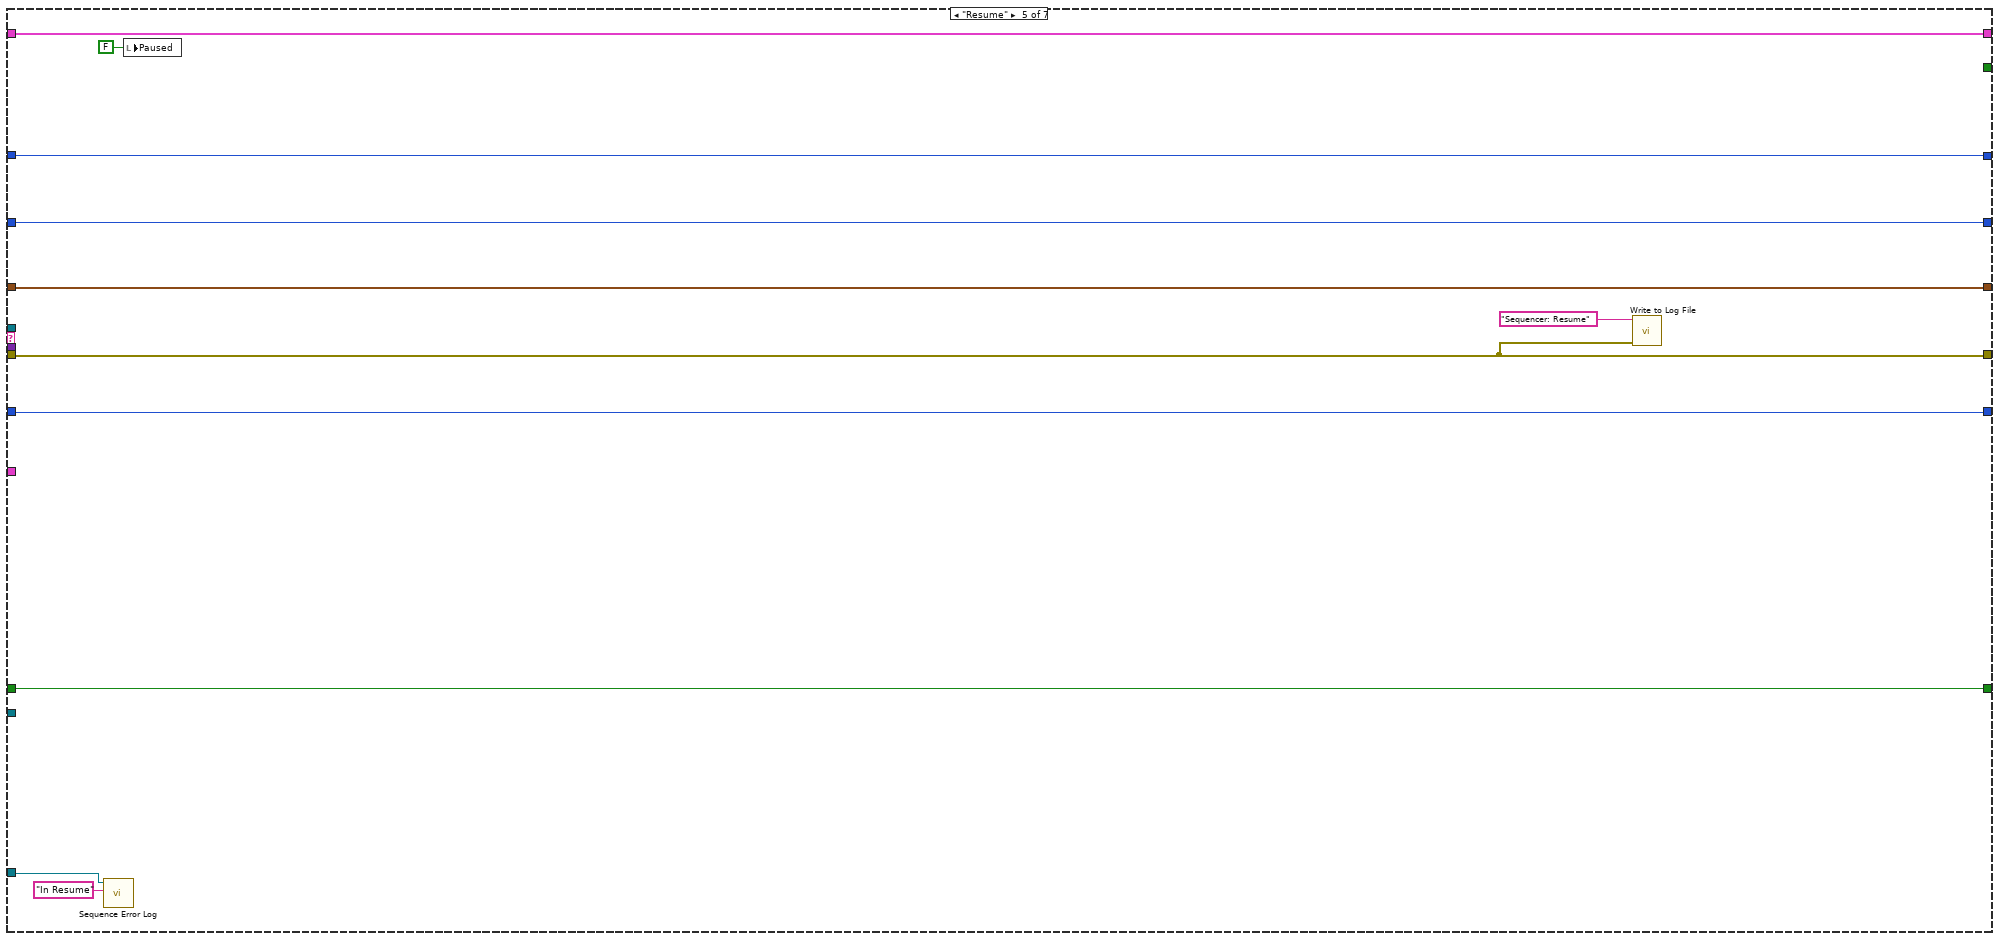
[diagram p14: hidden frame]
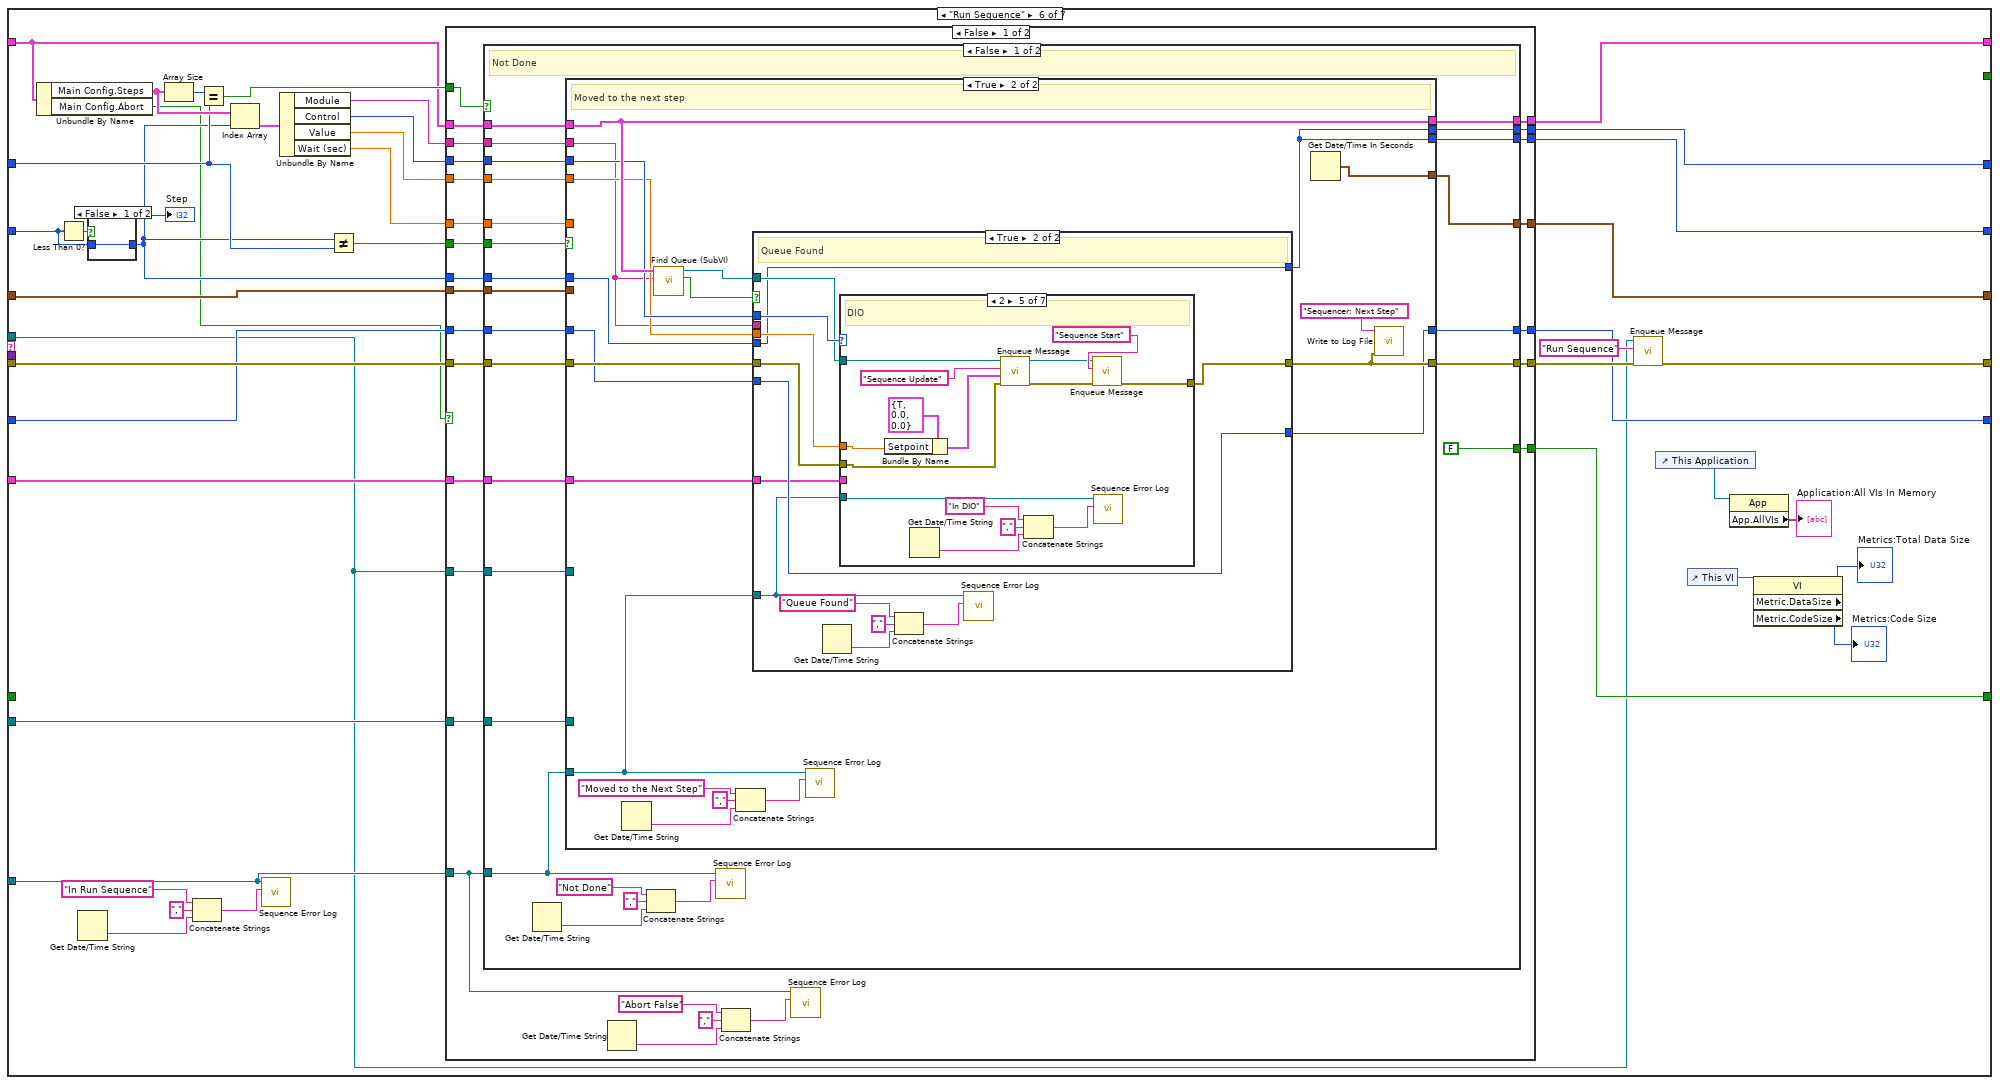
[diagram p15: hidden frame]
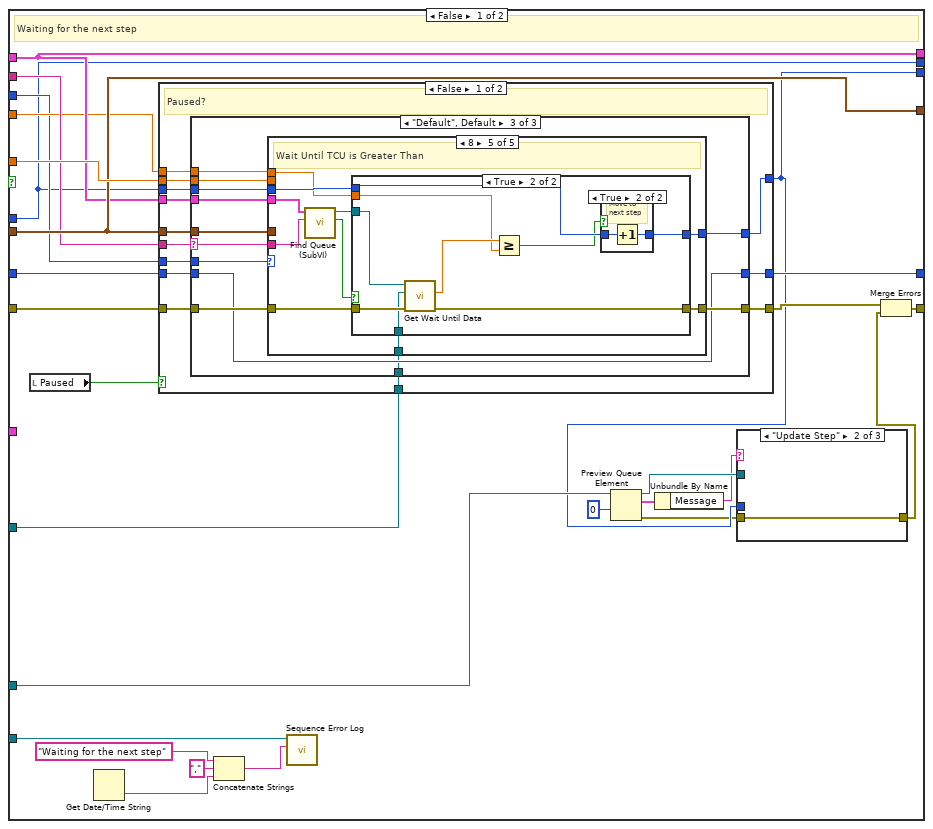
[diagram p16: hidden frame]
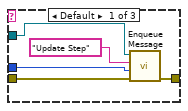
[diagram p17: hidden frame]
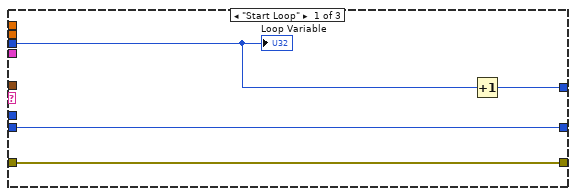
[diagram p19: hidden frame]
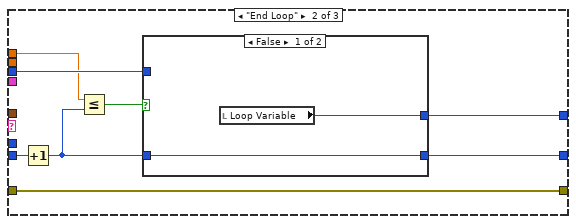
[diagram p20: hidden frame]
diagram:
  # "Loop Count"
  # "This step"
  # "Last Step"
  n1 = flat-sequence {
    tunnel: [w19] -> w14
    tunnel: [w31] -> w6
    tunnel: "error in (no error)" -> [w19]
    frame #0 {
      w37 = FALSE ("Paused")
      n2 = local write "Stop"(w37) -> ()
      n3 = local write "Done"(w37) -> ()
      n4 = local write "Paused"(w37) -> ()
      n5 = Get Date/Time String() -> (date string=w30:string, time string=w25:string)  [unwired: 3 in]
      n6 = Search and Replace String(replace all?=TRUE ("replace all? (F)"), input string=w30, search string="/", replace string="_" ("replace string (\"\")")) -> (result string=w21:string)  [unwired: 4 in, 3 out]
      n7 = Search and Replace String(replace all?=TRUE ("replace all? (F)"), input string=w25, search string=":", replace string="_" ("replace string (\"\")")) -> (result string=w20:string)  [unwired: 4 in, 3 out]
      n8 = Concatenate Strings("Sequence Log " ("string"), w21, w20) -> (w36:string)
      n9 = Build Path(base path=path "C:/Users/Public/Documents/Sequence Crash Error Log", name or relative path=w36) -> (appended path=w35:path)
      n10 = Open/Create/Replace File(file path (use dialog)=w35, operation (0:open)=T67."open or create") -> (refnum out=w31:refnum<file>, error out=→"error out 2":errorcluster)  [unwired: 4 in, 1 out]
    }
  }
  n11 = Unbundle By Name("Message Queues in") -> ("Sequence"=w17:refnum<queue>, "Sequence UI"=w8:refnum<queue>)
  n12 = call "Obtain Message Queue.vi"("name (unnamed)"="Sequence Loop") -> ("Message Queue"=w15:refnum<queue>)  [unwired: 9 in, 1 out]
  n13 = while {
    tunnel: w17 -> [w40]
    tunnel: w14 -> [w43]
    tunnel: [w44] -> w13
    tunnel: w15 -> [w39]
    tunnel: [w38] -> w3
    stop <- w41 stop-if-true
    n14 = call "Dequeue Message.vi"("error in (no error)"=w43, "Message Queue"=w40) -> ("error out"=w42:errorcluster, "Message Data"=w45:variant, "Message"=w46:string, "dup Message Queue"=w38:refnum<queue>)  [unwired: 6 in]
    n15 = case shown="\"Update Sequence\"" w46 {
      tunnel: w45 -> [_ _ _ _ w65 w70 w75]
      tunnel: w42 -> [w47 w54 w58 w63 w67 w72 w77]
      tunnel: [w47 w48 w57 w62 w66 w71 w76] -> w44
      tunnel: [_ _ w55 w60 _ _ _] -> w41
      tunnel: w39 -> [_ w52 w56 w61 w68 w73 w78]
      frame Default {
      }
      frame "Start Sequence" {
        n16 = call-poly "Enqueue Message.vi"("error in (no error)"=w54, "Message"="Send Settings", "Message Queue"=w52) -> ("error out"=w49:errorcluster, "dup Message Queue"=w51:refnum<queue>)  [unwired: 7 in]
        n17 = call-poly "Enqueue Message.vi"("error in (no error)"=w49, "Message"="Run Sequence", "Message Queue"=w51) -> ("error out"=w48:errorcluster)  [unwired: 7 in, 1 out]
      }
      frame "E-Stop", "Stop" {
        w55 = FALSE
        n18 = call-poly "Enqueue Message.vi"("error in (no error)"=w58, "Message"="Pause", "Message Queue"=w56) -> ("error out"=w57:errorcluster)  [unwired: 7 in, 1 out]
        "Stop" <- w55
      }
      frame "Exit" {
        w60 = TRUE
        n19 = call-poly "Enqueue Message.vi"("error in (no error)"=w63, "Message"="Exit", "Message Queue"=w61) -> ("error out"=w62:errorcluster)  [unwired: 7 in, 1 out]
        n20 = local write "Stop"(w60) -> ()
      }
      frame "Update Sequence" {
        n21 = call-poly "Enqueue Message.vi"("error in (no error)"=w67, "Message Data"=w65, "Message"="Update Sequence", "Message Queue"=w68) -> ("error out"=w66:errorcluster)  [unwired: 6 in, 1 out]
      }
      frame "Pause Sequence" {
        n22 = call-poly "Enqueue Message.vi"("error in (no error)"=w72, "Message Data"=w70, "Message"="Pause", "Message Queue"=w73) -> ("error out"=w71:errorcluster)  [unwired: 6 in, 1 out]
      }
      frame "Resume Sequence" {
        n23 = call-poly "Enqueue Message.vi"("error in (no error)"=w77, "Message Data"=w75, "Message"="Resume", "Message Queue"=w78) -> ("error out"=w76:errorcluster)  [unwired: 6 in, 1 out]
      }
    }
  }
  n24 = while {
    tunnel: w15 -> [w81]
    tunnel: w14 -> [w104]
    shift-right: [w101] -> _
    shift-left: _ -> [w91]
    tunnel: [w99] -> w11
    shift-right: [w94] -> _
    shift-left: -1 -> [w96]
    shift-right: [w93] -> _
    shift-left: _ -> [w95]
    shift-right: [w89] -> _
    shift-left: -1 -> [w90]
    shift-right: [w88] -> _
    shift-left: _ -> [w87]
    tunnel: w8 -> [w80]
    shift-right: [w86] -> _
    shift-left: 0 -> [w85]
    tunnel: w6 -> [w83]
    tunnel: T66 {"Auto?"=TRUE, "Manual Entry"=0.0, "Setpoint"=0.0} -> [w82]
    tunnel: [w81] -> w2
    tunnel: [w80] -> w1
    stop <- w98 stop-if-true
    n25 = call "Dequeue Message.vi"("error in (no error)"=w104, "timeout in ms (-1)"=1, "Message Queue"=w81) -> ("error out"=w100:errorcluster, "Message Data"=w102:variant, "Message"=w103:string, "dup Message Queue"=w92:refnum<queue>)  [unwired: 5 in]
    n26 = Wait (ms)(milliseconds to wait=u32 5) -> ()  [unwired: 1 out]
    n27 = case shown="\"Update Sequence\"" w103 {
      tunnel: w102 -> [_ w132 _ _ _ _ _]
      tunnel: [w114 w122 w141 w213 w224 w264 w711] -> w101
      tunnel: w100 -> [w113 w131 w135 w206 w217 w263 w710]
      tunnel: [w113 w124 w137 w206 w217 w252 w710] -> w99
      tunnel: [_ _ _ _ _ _ TRUE] -> w98
      tunnel: w91 -> [w114 _ w141 w213 w224 w246 w711]
      tunnel: w96 -> [w112 w129 _ w211 w222 w249 w709]
      tunnel: w95 -> [w111 w128 w142 w212 w223 w243 w708]
      tunnel: w90 -> [w109 w127 _ w209 w220 w255 w707]
      tunnel: [w112 w129 w139 w211 w222 w261 w709] -> w94
      tunnel: [w111 w128 w142 w212 w223 w258 w708] -> w93
      tunnel: w92 -> [_ _ _ _ _ w225 _]
      tunnel: [w109 w127 w139 w209 w220 w248 w707] -> w89
      tunnel: [w108 w126 FALSE w208 w219 w242 w706] -> w88
      tunnel: w87 -> [w108 w126 _ w208 w219 _ w706]
      tunnel: w80 -> [_ _ _ _ _ w240 _]
      tunnel: [w107 w123 w136 w205 w216 w239 w705] -> w86
      tunnel: w85 -> [w107 w123 w136 w205 w216 w238 w705]
      tunnel: w83 -> [w106 w115 w133 w203 w214 w232 w703]
      tunnel: w82 -> [_ _ _ _ _ w231 _]
      frame Default {
        n28 = call "Sequence Error Log.vi"("string"="In Default", "Byte Stream File in"=w106) -> ()  [unwired: 10 in]
        n29 = Wait (ms)(milliseconds to wait=u32 1000) -> ()  [unwired: 1 out]
      }
      frame "Update Sequence" {
        n30 = call "Sequence Error Log.vi"("string"="In Update Sequence", "Byte Stream File in"=w115) -> ()  [unwired: 10 in]
        n31 = Variant To Data(error in=w131, type="Input", Variant=w132) -> (data=w122:T1, error out=w124:errorcluster)
        "Output" <- w122
        n32 = Unbundle By Name(w122) -> ("Main Config.Pump Module Configs"=w121:T41[])
        n33 = Index Array(array=w121, index=0) -> (element=w119:T41)
        n34 = Unbundle By Name(w119) -> ("Process Name"=→"Process Name":string, "Queue Name"=→"Queue Name":string)
        n35 = call "Write to Log File.vi"("error in"=w124, "text"="Sequencer: Update") -> ()  [unwired: 9 in, 1 out]
      }
      frame "Send Settings" {
        w139 = -1
        n36 = Unbundle By Name(w141) -> ("Main Config.Steps"=w144:T54)
        n37 = call "Sequence Error Log.vi"("string"="In Send Settings", "Byte Stream File in"=w133) -> ()  [unwired: 10 in]
        n38 = for {
          tunnel: w144 -> [w153] mode=indexing
          tunnel: [w148] -> w143 mode=indexing
          tunnel: w135 -> [w150]
          tunnel: w141 -> [w147]
          n39 = Unbundle By Name(w153) -> ("Module"=w152:string, "Control"=w145:u16, "Value"=w154:dbl)
          n40 = call "Find Queue (SubVI).vi"("Module"=w152, "Input"=w147) -> ("Found?"=w151:bool, "Queue out"=w146:refnum<queue>)  [unwired: 8 in]
          n41 = case shown="0, Default" w145 {
            tunnel: [w188 w192 w196 w200] -> w149
            tunnel: w154 -> [w187 w191 w195 w199]
            frame 0, Default {
              n42 = Bundle By Name(cluster=T66 {"Auto?"=TRUE, "Manual Entry"=0.0, "Setpoint"=0.0}, "Auto?"=FALSE, "Manual Entry"=w187) -> (w188:T66)
            }
            frame 1 {
              n43 = Bundle By Name(cluster=T66 {"Auto?"=TRUE, "Manual Entry"=0.0, "Setpoint"=0.0}, "Auto?"=TRUE, "Setpoint"=w191) -> (w192:T66)
            }
            frame 5 {
              n44 = Bundle By Name(cluster=T66 {"Auto?"=TRUE, "Manual Entry"=0.0, "Setpoint"=0.0}, "Auto?"=TRUE, "Setpoint"=w195) -> (w196:T66)
            }
            frame 6 {
              n45 = Bundle By Name(cluster=T66 {"Auto?"=TRUE, "Manual Entry"=0.0, "Setpoint"=0.0}, "Auto?"=TRUE, "Setpoint"=w199) -> (w200:T66)
            }
          }
          n46 = case shown="True" w151 {
            tunnel: w150 -> [w155 w160]
            tunnel: w149 -> [_ w159]
            tunnel: [w155 w158] -> w148
            tunnel: w146 -> [_ w157]
            tunnel: w145 -> [_ w156]
            frame False {
            }
            frame True {
              n47 = case shown="6" w156 {
                tunnel: w160 -> [w165 w166 w170 w180]
                tunnel: w159 -> [w164 _ w169 w179]
                tunnel: [w162 w166 w168 w178] -> w158
                tunnel: w157 -> [w161 _ w167 w177]
                frame Default {
                  n48 = call-poly "Enqueue Message.vi"("error in (no error)"=w165, "Message Data"=w164, "Message"="Sequence Update", "Message Queue"=w161) -> ("error out"=w162:errorcluster)  [unwired: 6 in, 1 out]
                }
                frame 3, 4, 7, 8 {
                }
                frame 5 {
                  n49 = disable-structure shown="Disabled" {
                    disable-tunnel: w170 -> [w175 w176]
                    disable-tunnel: w169 -> [w174 _]
                    disable-tunnel: [w172 w176] -> w168
                    disable-tunnel: w167 -> [w171 _]
                    frame Disabled {
                      n50 = call-poly "Enqueue Message.vi"("error in (no error)"=w175, "Message Data"=w174, "Message"="Sequence Update Speed", "Message Queue"=w171) -> ("error out"=w172:errorcluster)  [unwired: 6 in, 1 out]
                    }
                    frame Enabled {
                    }
                  }
                }
                frame 6 {
                  n51 = disable-structure shown="Disabled" {
                    disable-tunnel: w180 -> [w185 w186]
                    disable-tunnel: w179 -> [w184 _]
                    disable-tunnel: [w182 w186] -> w178
                    disable-tunnel: w177 -> [w181 _]
                    frame Disabled {
                      n52 = call-poly "Enqueue Message.vi"("error in (no error)"=w185, "Message Data"=w184, "Message"="Sequence Update Temperature", "Message Queue"=w181) -> ("error out"=w182:errorcluster)  [unwired: 6 in, 1 out]
                    }
                    frame Enabled {
                    }
                  }
                }
              }
            }
          }
          "Intruction Cluster" <- w153
        }
        n53 = Merge Errors(w135, w143) -> (w137:errorcluster)
        n54 = call "Write to Log File.vi"("error in"=w137, "text"="Sequencer: Send Settings") -> ()  [unwired: 9 in, 1 out]
      }
      frame "Pause" {
        n55 = call "Sequence Error Log.vi"("string"="In Pause", "Byte Stream File in"=w203) -> ()  [unwired: 10 in]
        n56 = call "Write to Log File.vi"("error in"=w206, "text"="Sequencer: Pause") -> ()  [unwired: 9 in, 1 out]
        "Paused" <- TRUE ("Paused")
      }
      frame "Resume" {
        n57 = call "Sequence Error Log.vi"("string"="In Resume", "Byte Stream File in"=w214) -> ()  [unwired: 10 in]
        n58 = local write "Paused"(FALSE ("Paused")) -> ()
        n59 = call "Write to Log File.vi"("error in"=w217, "text"="Sequencer: Resume") -> ()  [unwired: 9 in, 1 out]
      }
      frame "Run Sequence" {
        n60 = Unbundle By Name(w246) -> ("Main Config.Steps"=w257:T54, "Main Config.Abort"=w237:bool)
        n61 = Less Than 0?(x=w249) -> (x < 0?=w250:bool)
        n62 = Get Date/Time String() -> (time string=w234:string)  [unwired: 3 in, 1 out]
        n63 = case shown="False" w250 {
          tunnel: [w701 0] -> w241
          tunnel: w249 -> [w701 _]
          frame False {
          }
          frame True {
          }
        }
        "Step" <- w241
        n64 = Array Size(array=w257) -> (size(s)=w256:i32)
        n65 = Concatenate Strings("In Run Sequence" ("string"), "," ("string"), w234) -> (w233:string)
        n66 = Equal?(x=w256, y=w255) -> (x = y?=w254:bool)
        n67 = Index Array(array=w257, index=w241) -> (element=w260:T55)
        n68 = call "Sequence Error Log.vi"("string"=w233, "Byte Stream File in"=w232) -> ()  [unwired: 10 in]
        n69 = Unbundle By Name(w260) -> ("Module"=w259:string, "Control"=w245:u16, "Value"=w244:dbl, "Wait (sec)"=w247:dbl)
        n70 = Not Equal?(x=w241, y=w255) -> (x != y?=w262:bool)
        n71 = case shown="False" w237 {
          tunnel: [w290 w692] -> w264
          tunnel: w263 -> [w289 w694]
          tunnel: w262 -> [w288 _]
          tunnel: [w287 w690] -> w261
          tunnel: w259 -> [w286 _]
          tunnel: [w285 w695] -> w258
          tunnel: w254 -> [w284 _]
          tunnel: [w283 w694] -> w253
          tunnel: [w282 w690] -> w248
          tunnel: w247 -> [w281 _]
          tunnel: w246 -> [w280 w692]
          tunnel: w245 -> [w279 _]
          tunnel: w244 -> [w278 _]
          tunnel: w243 -> [w277 w695]
          tunnel: [w276 TRUE] -> w242
          tunnel: w241 -> [w275 _]
          tunnel: w240 -> [w274 _]
          tunnel: [w273 0] -> w239
          tunnel: w238 -> [w272 _]
          tunnel: w232 -> [w267 w682]
          tunnel: w231 -> [w266 _]
          tunnel: w225 -> [w265 _]
          frame False {
            n72 = case shown="False" w284 {
              tunnel: [w315 w676] -> w290
              tunnel: w289 -> [w306 w670]
              tunnel: w280 -> [w314 w676]
              tunnel: [w313 w670] -> w283
              tunnel: w288 -> [w312 _]
              tunnel: w275 -> [w311 w674]
              tunnel: [w310 w674] -> w287
              tunnel: w286 -> [w309 _]
              tunnel: w281 -> [w308 _]
              tunnel: [w307 w673] -> w285
              tunnel: [w305 w674] -> w282
              tunnel: w279 -> [w304 _]
              tunnel: w278 -> [w303 _]
              tunnel: w277 -> [w302 w673]
              tunnel: [FALSE w672] -> w276
              tunnel: w274 -> [w300 _]
              tunnel: [w299 0] -> w273
              tunnel: w272 -> [w298 _]
              tunnel: w267 -> [w293 w664]
              tunnel: w266 -> [w292 _]
              tunnel: w265 -> [w291 _]
              frame False {
                # "Not Done"
                n73 = Get Date/Time String() -> (time string=w295:string)  [unwired: 3 in, 1 out]
                n74 = case shown="True" w312 {
                  tunnel: [w339 w522] -> w315
                  tunnel: w311 -> [w334 w512]
                  tunnel: w314 -> [w339 w522]
                  tunnel: [w332 w514] -> w313
                  tunnel: [w321 w511] -> w310
                  tunnel: w309 -> [w338 w513]
                  tunnel: w308 -> [w342 _]
                  tunnel: [w340 w516] -> w307
                  tunnel: w306 -> [w337 w519]
                  tunnel: [w334 w511] -> w305
                  tunnel: w304 -> [w335 w518]
                  tunnel: w303 -> [w336 w517]
                  tunnel: w302 -> [w340 _]
                  tunnel: w300 -> [w323 _]
                  tunnel: [w331 w509] -> w299
                  tunnel: w298 -> [w330 w510]
                  tunnel: w293 -> [w325 w504]
                  tunnel: w292 -> [_ w503]
                  tunnel: w291 -> [w324 _]
                  frame False {
                    # "Waiting for the next step"
                    n75 = local read "Paused"() -> (w341:bool)
                    n76 = Get Date/Time String() -> (time string=w327:string)  [unwired: 3 in, 1 out]
                    n77 = case shown="False" w341 {
                      tunnel: [w362 w502] -> w321
                      tunnel: w334 -> [w361 w502]
                      tunnel: w342 -> [w360 _]
                      tunnel: w340 -> [w359 _]
                      tunnel: w335 -> [w358 _]
                      tunnel: w339 -> [w357 _]
                      tunnel: w338 -> [w353 _]
                      tunnel: w337 -> [w356 w501]
                      tunnel: [w355 w501] -> w333
                      tunnel: w336 -> [w354 _]
                      tunnel: [w352 w500] -> w331
                      tunnel: w330 -> [w351 w500]
                      tunnel: w324 -> [w350 _]
                      frame False {
                        # "Paused?"
                        n78 = case shown="\"Default\", Default" w353 {
                          selector: w353 -> [_ _ w382]
                          tunnel: [w364 w374 w391] -> w362
                          tunnel: w361 -> [w365 w372 w390]
                          tunnel: w360 -> [_ _ w389]
                          tunnel: w359 -> [_ _ w388]
                          tunnel: w358 -> [_ _ w387]
                          tunnel: w357 -> [_ _ w386]
                          tunnel: w356 -> [w366 w373 w385]
                          tunnel: [w366 w373 w384] -> w355
                          tunnel: w354 -> [_ w370 w383]
                          tunnel: [w363 w369 w381] -> w352
                          tunnel: w351 -> [w363 w368 w381]
                          tunnel: w350 -> [_ _ w380]
                          frame "Start Loop" {
                            n79 = Increment(x=w365) -> (x+1=w364:u32)
                            "Loop Variable" <- w365
                          }
                          frame "End Loop" {
                            n80 = Increment(x=w368) -> (x+1=w367:i32)
                            n81 = Less Or Equal?(x=w370, y=w367) -> (x <= y?=w371:bool)
                            n82 = case shown="False" w371 {
                              tunnel: [w376 w378] -> w374
                              tunnel: w372 -> [_ w379]
                              tunnel: [w375 w377] -> w369
                              tunnel: w367 -> [w375 w377]
                              frame False {
                                n83 = local read "Loop Variable"() -> (w376:u32)
                              }
                              frame True {
                                n84 = Increment(x=w379) -> (x+1=w378:u32)
                              }
                            }
                          }
                          frame "Default", Default {
                            n85 = case shown="8" w387 {
                              tunnel: [w396 w412 w436 w460 w484] -> w391
                              tunnel: w390 -> [w395 w411 w435 w459 w483]
                              tunnel: w389 -> [w394 _ _ _ _]
                              tunnel: w388 -> [w393 _ _ _ _]
                              tunnel: w386 -> [_ w410 w434 w458 w482]
                              tunnel: w382 -> [_ w409 w433 w457 w481]
                              tunnel: w385 -> [w392 w406 w430 w454 w478]
                              tunnel: [w392 w405 w429 w453 w477] -> w384
                              tunnel: w383 -> [_ w404 w428 w452 w476]
                              tunnel: w380 -> [_ w403 w427 w451 w475]
                              frame 0..2, 5, 6, Default {
                                n86 = Get Date/Time In Seconds() -> (seconds since 1Jan1904=w399:timestamp)
                                n87 = Subtract(x=w399, y=w393) -> (x-y=w397:dbl)
                                n88 = Greater Or Equal?(x=w397, y=w394) -> (x >= y?=w398:bool)
                                n89 = case shown="True" w398 {
                                tunnel: w395 -> [w400 w402]
                                tunnel: [w400 w401] -> w396
                                frame False {
                                }
                                frame True {
                                # "Move to next step"
                                n90 = Increment(x=w402) -> (x+1=w401:u32)
                                }
                                }
                              }
                              frame 3 {
                                # "Wait Until Less Than"
                                n91 = call "Find Queue (SubVI).vi"("Module"=w409, "Input"=w410) -> ("Found?"=w408:bool, "Queue out"=w407:refnum<queue>)  [unwired: 8 in]
                                n92 = case shown="True" w408 {
                                tunnel: [w414 w423] -> w412
                                tunnel: w411 -> [w414 w422]
                                tunnel: w407 -> [_ w421]
                                tunnel: w406 -> [w413 w420]
                                tunnel: [w413 w419] -> w405
                                tunnel: w404 -> [_ w417]
                                tunnel: w403 -> [_ w415]
                                frame False {
                                # "Error"
                                }
                                frame True {
                                n93 = call "Get Wait Until Data.vi"("error in (no error)"=w420, "Sequence Data Queue"=w415, "Queue in"=w421) -> ("error out"=w419:errorcluster, "Data"=w418:dbl)  [unwired: 7 in]
                                n94 = Less Or Equal?(x=w418, y=w417) -> (x <= y?=w416:bool)
                                n95 = case shown="True" w416 {
                                tunnel: w422 -> [w424 w426]
                                tunnel: [w424 w425] -> w423
                                frame False {
                                }
                                frame True {
                                # "Move to next step"
                                n96 = Increment(x=w426) -> (x+1=w425:u32)
                                }
                                }
                                }
                                }
                              }
                              frame 4 {
                                # "Wait Until Greater Than"
                                n97 = call "Find Queue (SubVI).vi"("Module"=w433, "Input"=w434) -> ("Found?"=w432:bool, "Queue out"=w431:refnum<queue>)  [unwired: 8 in]
                                n98 = case shown="True" w432 {
                                tunnel: [w438 w447] -> w436
                                tunnel: w435 -> [w438 w446]
                                tunnel: w431 -> [_ w445]
                                tunnel: w430 -> [w437 w444]
                                tunnel: [w437 w443] -> w429
                                tunnel: w428 -> [_ w441]
                                tunnel: w427 -> [_ w439]
                                frame False {
                                # "Error"
                                }
                                frame True {
                                n99 = call "Get Wait Until Data.vi"("error in (no error)"=w444, "Sequence Data Queue"=w439, "Queue in"=w445) -> ("error out"=w443:errorcluster, "Data"=w442:dbl)  [unwired: 7 in]
                                n100 = Greater Or Equal?(x=w442, y=w441) -> (x >= y?=w440:bool)
                                n101 = case shown="True" w440 {
                                tunnel: w446 -> [w448 w450]
                                tunnel: [w448 w449] -> w447
                                frame False {
                                }
                                frame True {
                                # "Move to next step"
                                n102 = Increment(x=w450) -> (x+1=w449:u32)
                                }
                                }
                                }
                                }
                              }
                              frame 7 {
                                # "Wait Until TCU is Less Than"
                                n103 = call "Find Queue (SubVI).vi"("Module"=w457, "Input"=w458) -> ("Found?"=w456:bool, "Queue out"=w455:refnum<queue>)  [unwired: 8 in]
                                n104 = case shown="True" w456 {
                                tunnel: [w462 w471] -> w460
                                tunnel: w459 -> [w462 w470]
                                tunnel: w455 -> [_ w469]
                                tunnel: w454 -> [w461 w468]
                                tunnel: [w461 w467] -> w453
                                tunnel: w452 -> [_ w465]
                                tunnel: w451 -> [_ w463]
                                frame False {
                                # "Error"
                                }
                                frame True {
                                n105 = call "Get Wait Until Data.vi"("error in (no error)"=w468, "Sequence Data Queue"=w463, "Queue in"=w469) -> ("error out"=w467:errorcluster, "Data"=w466:dbl)  [unwired: 7 in]
                                n106 = Less Or Equal?(x=w466, y=w465) -> (x <= y?=w464:bool)
                                n107 = case shown="True" w464 {
                                tunnel: w470 -> [w472 w474]
                                tunnel: [w472 w473] -> w471
                                frame False {
                                }
                                frame True {
                                # "Move to next step"
                                n108 = Increment(x=w474) -> (x+1=w473:u32)
                                }
                                }
                                }
                                }
                              }
                              frame 8 {
                                # "Wait Until TCU is Greater Than"
                                n109 = call "Find Queue (SubVI).vi"("Module"=w481, "Input"=w482) -> ("Found?"=w480:bool, "Queue out"=w479:refnum<queue>)  [unwired: 8 in]
                                n110 = case shown="True" w480 {
                                tunnel: [w486 w495] -> w484
                                tunnel: w483 -> [w486 w494]
                                tunnel: w479 -> [_ w493]
                                tunnel: w478 -> [w485 w492]
                                tunnel: [w485 w491] -> w477
                                tunnel: w476 -> [_ w489]
                                tunnel: w475 -> [_ w487]
                                frame False {
                                # "Error"
                                }
                                frame True {
                                n111 = call "Get Wait Until Data.vi"("error in (no error)"=w492, "Sequence Data Queue"=w487, "Queue in"=w493) -> ("error out"=w491:errorcluster, "Data"=w490:dbl)  [unwired: 7 in]
                                n112 = Greater Or Equal?(x=w490, y=w489) -> (x >= y?=w488:bool)
                                n113 = case shown="True" w488 {
                                tunnel: w494 -> [w496 w498]
                                tunnel: [w496 w497] -> w495
                                frame False {
                                }
                                frame True {
                                # "Move to next step"
                                n114 = Increment(x=w498) -> (x+1=w497:u32)
                                }
                                }
                                }
                                }
                              }
                            }
                          }
                        }
                      }
                      frame True {
                        # "Paused?"
                        n115 = Wait (ms)(milliseconds to wait=u32 50) -> ()  [unwired: 1 out]
                      }
                    }
                    n116 = Concatenate Strings("Waiting for the next step" ("string"), "," ("string"), w327) -> (w326:string)
                    n117 = call "Sequence Error Log.vi"("string"=w326, "Byte Stream File in"=w325) -> ()  [unwired: 10 in]
                    n118 = Preview Queue Element(queue=w323, timeout in ms (-1)=0) -> (queue out=w320:refnum<queue>, element=w318:T68, error out=w316:errorcluster)  [unwired: 1 in, 1 out]
                    n119 = Unbundle By Name(w318) -> ("Message"=w317:string)
                    n120 = case shown="\"Update Step\"" w317 {
                      tunnel: w321 -> [w343 _ _]
                      tunnel: w320 -> [w344 _ _]
                      tunnel: [w345 w348 w349] -> w319
                      tunnel: w316 -> [w346 w348 w349]
                      frame Default {
                        n121 = call-poly "Enqueue Message.vi"("error in (no error)"=w346, "Message Data"=w343, "Message"="Update Step", "Message Queue"=w344) -> ("error out"=w345:errorcluster)  [unwired: 6 in, 1 out]
                      }
                      frame "Update Step" {
                      }
                      frame "Exit" {
                      }
                    }
                    n122 = Merge Errors(w333, w319) -> (w332:errorcluster)
                  }
                  frame True {
                    # "Moved to the next step"
                    n123 = Get Date/Time String() -> (time string=w506:string)  [unwired: 3 in, 1 out]
                    n124 = call "Find Queue (SubVI).vi"("Module"=w513, "Input"=w522) -> ("Found?"=w521:bool, "Queue out"=w520:refnum<queue>)  [unwired: 8 in]
                    n125 = Concatenate Strings("Moved to the Next Step" ("string"), "," ("string"), w506) -> (w505:string)
                    n126 = case shown="True" w521 {
                      tunnel: w520 -> [_ w565]
                      tunnel: w519 -> [w534 w564]
                      tunnel: [w533 w563] -> w514
                      tunnel: w518 -> [_ w567]
                      tunnel: w517 -> [w529 w566]
                      tunnel: w513 -> [w535 _]
                      tunnel: w512 -> [w532 w562]
                      tunnel: [w531 w562] -> w511
                      tunnel: w510 -> [w530 w561]
                      tunnel: [w528 w561] -> w509
                      tunnel: w504 -> [w523 w556]
                      tunnel: w503 -> [_ w555]
                      frame False {
                        # "Queue not found. ERROR"
                        n127 = Get Date/Time String() -> (time string=w525:string)  [unwired: 3 in, 1 out]
                        n128 = case shown="\"End Loop\"" w535 {
                          tunnel: [w538 w545 w554] -> w533
                          tunnel: w534 -> [w538 w545 w554]
                          tunnel: w532 -> [w537 w541 w553]
                          tunnel: [w537 w546 w553] -> w531
                          tunnel: w530 -> [w536 w543 w552]
                          tunnel: w529 -> [_ w544 _]
                          tunnel: [w536 w540 w552] -> w528
                          frame "Start Loop" {
                            n129 = local write "Loop Variable"(w537) -> ()
                          }
                          frame "End Loop" {
                            n130 = Increment(x=w543) -> (x+1=w539:i32)
                            n131 = Less Or Equal?(x=w544, y=w539) -> (x <= y?=w542:bool)
                            n132 = case shown="True" w542 {
                              tunnel: [w548 w550] -> w546
                              tunnel: w541 -> [_ w551]
                              tunnel: [w547 0] -> w540
                              tunnel: w539 -> [w547 _]
                              frame False {
                                n133 = local read "Loop Variable"() -> (w548:u32)
                              }
                              frame True {
                                n134 = Increment(x=w551) -> (x+1=w550:u32)
                              }
                            }
                          }
                          frame "Default", Default {
                            # "Error"
                          }
                        }
                        n135 = Concatenate Strings("Queue Not Found" ("string"), "," ("string"), w525) -> (w524:string)
                        n136 = call "Sequence Error Log.vi"("string"=w524, "Byte Stream File in"=w523) -> ()  [unwired: 10 in]
                      }
                      frame True {
                        # "Queue Found"
                        n137 = Get Date/Time String() -> (time string=w558:string)  [unwired: 3 in, 1 out]
                        n138 = case shown="2" w567 {
                          tunnel: w566 -> [w581 w598 w613 w629 w644 _ _]
                          tunnel: w565 -> [w579 w595 w610 w626 w642 _ w660]
                          tunnel: w564 -> [w577 w594 w609 w625 w643 w652 w659]
                          tunnel: [w573 w590 w605 w621 w637 w652 w658] -> w563
                          tunnel: w556 -> [w568 w585 w600 w616 w632 w647 w653]
                          tunnel: w555 -> [_ w584 _ _ _ _ _]
                          frame 0 {
                            # "Manual"
                            n139 = Get Date/Time String() -> (time string=w570:string)  [unwired: 3 in, 1 out]
                            n140 = Bundle By Name(cluster=T66 {"Auto?"=TRUE, "Manual Entry"=0.0, "Setpoint"=0.0}, "Auto?"=FALSE, "Manual Entry"=w581) -> (w578:T66)
                            n141 = Concatenate Strings("In Manual" ("string"), "," ("string"), w570) -> (w569:string)
                            n142 = call-poly "Enqueue Message.vi"("error in (no error)"=w577, "Message Data"=w578, "Message"="Sequence Update", "Message Queue"=w579) -> ("error out"=w575:errorcluster, "dup Message Queue"=w576:refnum<queue>)  [unwired: 6 in]
                            n143 = call "Sequence Error Log.vi"("string"=w569, "Byte Stream File in"=w568) -> ()  [unwired: 10 in]
                            n144 = call-poly "Enqueue Message.vi"("error in (no error)"=w575, "Message"="Sequence Start", "Message Queue"=w576) -> ("error out"=w573:errorcluster)  [unwired: 7 in, 1 out]
                          }
                          frame 1 {
                            # "Auto"
                            n145 = Get Date/Time String() -> (time string=w587:string)  [unwired: 3 in, 1 out]
                            n146 = Bundle By Name(cluster=w584, "Auto?"=TRUE, "Setpoint"=w598) -> (w596:T66)
                            n147 = Concatenate Strings("In Auto" ("string"), "," ("string"), w587) -> (w586:string)
                            n148 = call-poly "Enqueue Message.vi"("error in (no error)"=w594, "Message Data"=w596, "Message"="Sequence Update", "Message Queue"=w595) -> ("error out"=w592:errorcluster, "dup Message Queue"=w591:refnum<queue>)  [unwired: 6 in]
                            n149 = call "Sequence Error Log.vi"("string"=w586, "Byte Stream File in"=w585) -> ()  [unwired: 10 in]
                            n150 = call-poly "Enqueue Message.vi"("error in (no error)"=w592, "Message"="Sequence Start", "Message Queue"=w591) -> ("error out"=w590:errorcluster)  [unwired: 7 in, 1 out]
                          }
                          frame 5 {
                            # "Update TCU Speed"
                            n151 = Get Date/Time String() -> (time string=w602:string)  [unwired: 3 in, 1 out]
                            n152 = Bundle By Name(cluster=T66 {"Auto?"=TRUE, "Manual Entry"=0.0, "Setpoint"=0.0}, "Auto?"=TRUE, "Setpoint"=w613) -> (w611:T66)
                            n153 = Concatenate Strings("Update TCU Speed" ("string"), "," ("string"), w602) -> (w601:string)
                            n154 = call-poly "Enqueue Message.vi"("error in (no error)"=w609, "Message Data"=w611, "Message"="Sequence Update Speed", "Message Queue"=w610) -> ("error out"=w607:errorcluster, "dup Message Queue"=w606:refnum<queue>)  [unwired: 6 in]
                            n155 = call "Sequence Error Log.vi"("string"=w601, "Byte Stream File in"=w600) -> ()  [unwired: 10 in]
                            n156 = call-poly "Enqueue Message.vi"("error in (no error)"=w607, "Message"="Sequence Start", "Message Queue"=w606) -> ("error out"=w605:errorcluster)  [unwired: 7 in, 1 out]
                          }
                          frame 6 {
                            # "Update TCU Tempurature"
                            n157 = Get Date/Time String() -> (time string=w618:string)  [unwired: 3 in, 1 out]
                            n158 = Bundle By Name(cluster=T66 {"Auto?"=TRUE, "Manual Entry"=0.0, "Setpoint"=0.0}, "Auto?"=TRUE, "Setpoint"=w629) -> (w627:T66)
                            n159 = Concatenate Strings("In Update TCU Temp" ("string"), "," ("string"), w618) -> (w617:string)
                            n160 = call-poly "Enqueue Message.vi"("error in (no error)"=w625, "Message Data"=w627, "Message"="Sequence Update Temperature", "Message Queue"=w626) -> ("error out"=w623:errorcluster, "dup Message Queue"=w622:refnum<queue>)  [unwired: 6 in]
                            n161 = call "Sequence Error Log.vi"("string"=w617, "Byte Stream File in"=w616) -> ()  [unwired: 10 in]
                            n162 = call-poly "Enqueue Message.vi"("error in (no error)"=w623, "Message"="Sequence Start", "Message Queue"=w622) -> ("error out"=w621:errorcluster)  [unwired: 7 in, 1 out]
                          }
                          frame 2 {
                            # "DIO"
                            n163 = Bundle By Name(cluster=T66 {"Auto?"=TRUE, "Manual Entry"=0.0, "Setpoint"=0.0}, "Setpoint"=w644) -> (w641:T66)
                            n164 = Get Date/Time String() -> (time string=w634:string)  [unwired: 3 in, 1 out]
                            n165 = call-poly "Enqueue Message.vi"("error in (no error)"=w643, "Message Data"=w641, "Message"="Sequence Update", "Message Queue"=w642) -> ("error out"=w638:errorcluster, "dup Message Queue"=w639:refnum<queue>)  [unwired: 6 in]
                            n166 = Concatenate Strings("In DIO" ("string"), "," ("string"), w634) -> (w633:string)
                            n167 = call-poly "Enqueue Message.vi"("error in (no error)"=w638, "Message"="Sequence Start", "Message Queue"=w639) -> ("error out"=w637:errorcluster)  [unwired: 7 in, 1 out]
                            n168 = call "Sequence Error Log.vi"("string"=w633, "Byte Stream File in"=w632) -> ()  [unwired: 10 in]
                          }
                          frame 3, 4 {
                            # "Wait until"
                            n169 = Get Date/Time String() -> (time string=w649:string)  [unwired: 3 in, 1 out]
                            n170 = Concatenate Strings("In Wait Until" ("string"), "," ("string"), w649) -> (w648:string)
                            n171 = call "Sequence Error Log.vi"("string"=w648, "Byte Stream File in"=w647) -> ()  [unwired: 10 in]
                          }
                          frame Default {
                            n172 = Get Date/Time String() -> (time string=w655:string)  [unwired: 3 in, 1 out]
                            n173 = call-poly "Enqueue Message.vi"("error in (no error)"=w659, "Message"="Sequence Start", "Message Queue"=w660) -> ("error out"=w658:errorcluster)  [unwired: 7 in, 1 out]
                            n174 = Concatenate Strings("In Default" ("string"), "," ("string"), w655) -> (w654:string)
                            n175 = call "Sequence Error Log.vi"("string"=w654, "Byte Stream File in"=w653) -> ()  [unwired: 10 in]
                          }
                        }
                        n176 = Concatenate Strings("Queue Found" ("string"), "," ("string"), w558) -> (w557:string)
                        n177 = call "Sequence Error Log.vi"("string"=w557, "Byte Stream File in"=w556) -> ()  [unwired: 10 in]
                      }
                    }
                    n178 = call "Sequence Error Log.vi"("string"=w505, "Byte Stream File in"=w504) -> ()  [unwired: 10 in]
                    n179 = Get Date/Time In Seconds() -> (seconds since 1Jan1904=w516:timestamp)
                    n180 = call "Write to Log File.vi"("error in"=w514, "text"="Sequencer: Next Step") -> ()  [unwired: 9 in, 1 out]
                  }
                }
                n181 = Concatenate Strings("Not Done" ("string"), "," ("string"), w295) -> (w294:string)
                n182 = call "Sequence Error Log.vi"("string"=w294, "Byte Stream File in"=w293) -> ()  [unwired: 10 in]
              }
              frame True {
                w672 = TRUE
                # "This VI closes the Command Log File"
                # "Done"
                n183 = Get Date/Time String() -> (time string=w666:string)  [unwired: 3 in, 1 out]
                n184 = Wait (ms)(milliseconds to wait=u32 100) -> ()  [unwired: 1 out]
                n185 = Concatenate Strings("Done" ("string"), "," ("string"), w666) -> (w662:string)
                n186 = flat-sequence {
                  tunnel: w664 -> [w677]
                  tunnel: [w677] -> w663
                  tunnel: w662 -> [w678]
                  tunnel: [w680] -> w665
                  tunnel: w663 -> [w680]
                  tunnel: w665 -> [w681]
                  frame #0 {
                    n187 = call "Sequence Error Log.vi"("string"=w678, "Byte Stream File in"=w677) -> ()  [unwired: 10 in]
                  }
                  frame #1 {
                    n188 = Wait (ms)(milliseconds to wait=u32 3000) -> ()  [unwired: 1 out]
                  }
                  frame #2 {
                    n189 = Close File(refnum=w681) -> ()  [unwired: 1 in, 2 out]
                  }
                }
                n190 = call "Write to Log File.vi"("error in"=w670, "text"="Sequencer: Done") -> ()  [unwired: 9 in, 1 out]
                "Done" <- w672
              }
            }
            n191 = Get Date/Time String() -> (time string=w269:string)  [unwired: 3 in, 1 out]
            n192 = Concatenate Strings("Abort False" ("string"), "," ("string"), w269) -> (w268:string)
            n193 = call "Sequence Error Log.vi"("string"=w268, "Byte Stream File in"=w267) -> ()  [unwired: 10 in]
          }
          frame True {
            n194 = Get Date/Time String() -> (time string=w686:string)  [unwired: 3 in, 1 out]
            n195 = Concatenate Strings("Abort True" ("string"), "," ("string"), w686) -> (w683:string)
            n196 = flat-sequence {
              tunnel: [w696] -> _
              tunnel: [w696] -> w685
              tunnel: w683 -> [w697]
              tunnel: w682 -> [w696]
              tunnel: [w699] -> w684
              tunnel: w685 -> [w699]
              tunnel: w684 -> [w700]
              frame #0 {
                n197 = call "Sequence Error Log.vi"("string"=w697, "Byte Stream File in"=w696) -> ()  [unwired: 10 in]
              }
              frame #1 {
                n198 = Wait (ms)(milliseconds to wait=u32 3000) -> ()  [unwired: 1 out]
              }
              frame #2 {
                n199 = Close File(refnum=w700) -> ()  [unwired: 1 in, 2 out]
              }
            }
            n200 = Unbundle By Name(w692) -> ("Main Config.Steps"=w691:T54)
            n201 = Array Size(array=w691) -> (size(s)=w690:i32)
          }
        }
        n202 = call-poly "Enqueue Message.vi"("error in (no error)"=w253, "Message"="Run Sequence", "Message Queue"=w225) -> ("error out"=w252:errorcluster)  [unwired: 7 in, 1 out]
        n203 = control-ref of="This Application"() -> (w230:refnum<vi>)
        n204 = control-ref of="This VI"() -> (w228:refnum<vi>)
        n205 = property class="App"(reference=w230) -> ("App.AllVIs"=→"Application:All VIs In Memory":string[])  [unwired: 1 in, 2 out]
        n206 = property class="VI"(reference=w228) -> ("Metric.DataSize"=→"Metrics:Total Data Size":u32, "Metric.CodeSize"=→"Metrics:Code Size":u32)  [unwired: 1 in, 2 out]
      }
      frame "Exit" {
        n207 = call "Sequence Error Log.vi"("string"="In Exit", "Byte Stream File in"=w703) -> ()  [unwired: 10 in]
      }
    }
  }
  n208 = Release Queue(queue=w3) -> ()  [unwired: 2 in, 3 out]
  n209 = Merge Errors(w13, w11) -> (→"error out":errorcluster)
  n210 = Release Queue(queue=w2) -> ()  [unwired: 2 in, 3 out]
  n211 = Release Queue(queue=w1) -> ()  [unwired: 2 in, 3 out]
